vi "ABR-CPMR.vi"() -> ()   [LabVIEW 2014]
uses:
  <vilib>/DAQmx/create/channels.llb/DAQmx Create Channel (AI-Voltage-Basic).vi
  <vilib>/DAQmx/configure/trigger.llb/DAQmx Start Trigger (Digital Edge).vi
  <vilib>/DAQmx/create/channels.llb/DAQmx Create Channel (AO-Voltage-Basic).vi
  <vilib>/DAQmx/configure/timing.llb/DAQmx Timing (Sample Clock).vi
  <vilib>/DAQmx/write.llb/DAQmx Write (Analog Wfm 1Chan NSamp).vi
  <vilib>/DAQmx/read.llb/DAQmx Read (Analog Wfm 1Chan NSamp).vi
  <vilib>/measure/NI_MABase.lvlib
  <resource>/objmgr/daqmx.rc
panel:
  out "Averaged Acq Graph":waveform(dbl)(graph)
  out "C settings str":string[][](array[string])
  out "WN settings str":string[][](array[string])
  out "PT settings str":string[][](array[string])
  in  "Stop!":bool
  out "Expinfo words":string[](array[string])
  out "counter 2":i32
  out "First file array":bool[](array[boolean])
  out "Current test":i32(knob) scale=0.0..10.0
  out "Delay duration (ms)":dbl[](array[numeric])
  out "Stimulus duration (ms)":dbl[](array[numeric])
  out "Signal duration (ms)":dbl[](array[numeric])
  out "End of test":bool
  out "Stim file name":string[](array[string])
  out "Date_Time":string
  out "Main file name":string[](array[string])
  out "Fs":string
  out "File path str":string
  in  "Subject ID":string
  out "Expinfo name":string[](array[string])
  out "File name":string[](array[string])
  in  "File path":path
  in  "User name":string
  out "Group array settings":dbl[][](array[numeric])
  out "counter":i32
  in  "Start!":bool
  in  "Output Channel":tag="PXI1Slot6/ao0"
  out "Acquisition Graph":waveform(dbl)(graph)
  in  "Input Channel":tag="PXI1Slot6/ai0"
  out "Fs (#S/s)":dbl
  out "Stimulus Graph":waveform(dbl)(graph)
  out "iteration2":i32
  in  "Sampling info":cluster{"Fs (#S/s)":dbl, "#S":dbl}={"Fs (#S/s)"=100000.0, "#S"=200000.0}
  out "Protocol list":string[](array[string])
  out "Protocol array settings":dbl[][](array[numeric])
  out "C settings":dbl[](array[numeric])
  out "WN settings":dbl[](array[numeric])
  in  "Type of stimulus":u16(ring)=3 items=["Pure Tones", "White Noise", "Clic", "Choose..."]
  out "C words":string[](array[string])
  out "WN words":string[](array[string])
  out "iteration":i32
  in  "How many tests?":i32(slide)=1 scale=0.0..10.0
  out "PT words":string[](array[string])
  out "PT settings":dbl[](array[numeric])
  out "Tab Control":enum32{"Pure Tones", "White Noise", "Clic"}(tab)
  in  "Frequency (Hz)":u16(ring)=500 items=["500"=500, "1k"=1000, "2k"=2000, "4k"=4000, "8k"=8000, "16k"=16000, "32k"=32000, "40k"=40000]
  in  "Stimulation freq (stim/sec)":i32=20
  in  "Add Button":bool
  in  "Amplitude (dB SPL)":dbl=10.0 min=10.0 max=90.0 step=10.0
  in  "# Repetitions":u16(ring)=1000 items=["500"=500, "1000"=1000, "1500"=1500, "2000"=2000]
  in  "Amplitude (dB SPL)":dbl=30.0 min=10.0 max=90.0 step=10.0
  in  "Stimulation freq (stim/sec)":i32=20
  in  "Add Button":bool
  in  "# Repetitions":u16(ring)=1000 items=["500"=500, "1000"=1000, "1500"=1500, "2000"=2000]
  in  "Add Button":bool
  in  "Amplitude (dB SPL)":dbl=10.0 min=10.0 max=90.0 step=10.0
  in  "Stimulation freq (stim/sec)":i32=20
  in  "# Repetitions":u16(ring)=1000 items=["500"=500, "1000"=1000, "1500"=1500, "2000"=2000]
  # "Protocol list:"
  # "User, Subject and File settings:"
  # "Protocol settings:"
  # "1"
  # "(without spaces)"
  # "(without spaces)"
  # "4"
  # "(without spaces)"
  # "5"
  # "2"
  # "Choose channels:"
  # "6"
  # "3"
  # "Select sample rate:"
  # "Copyright 2016 División de Ciencias e Ingenierías, Campus León,\nUniversidad de Guanajuato\nPor: Cecilia Paulina Mares Román <cecypau.mr@gmail.com>"
  # "8"
  # "7"
  # "7"
  # "7"
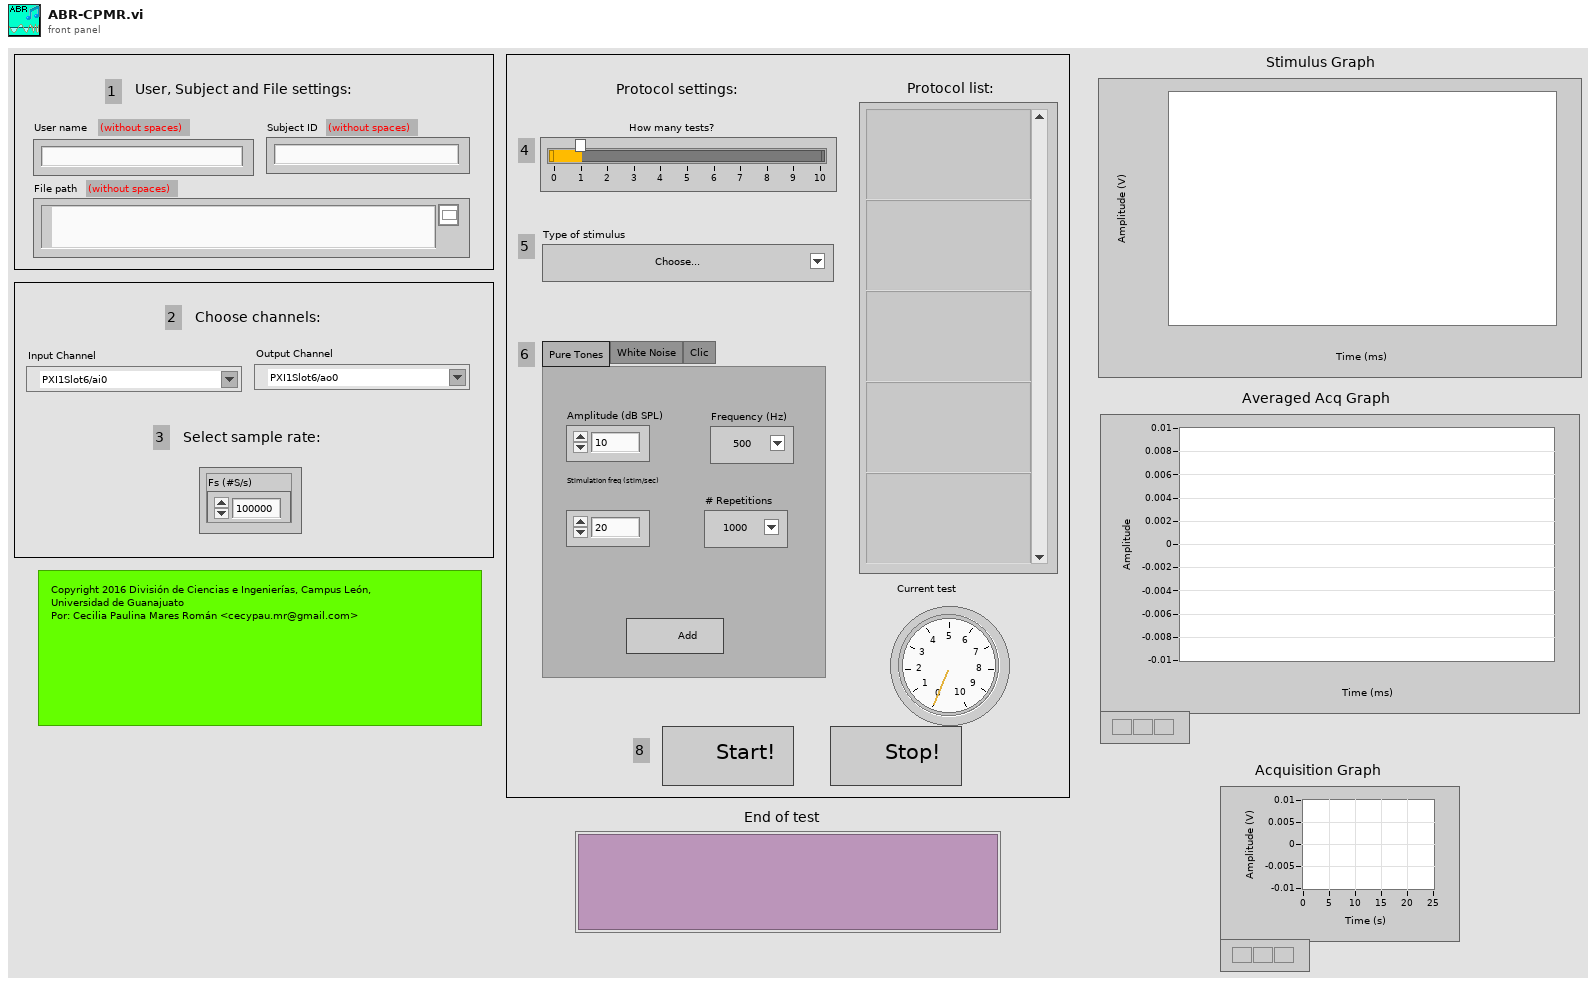
[diagram p1: front panel]
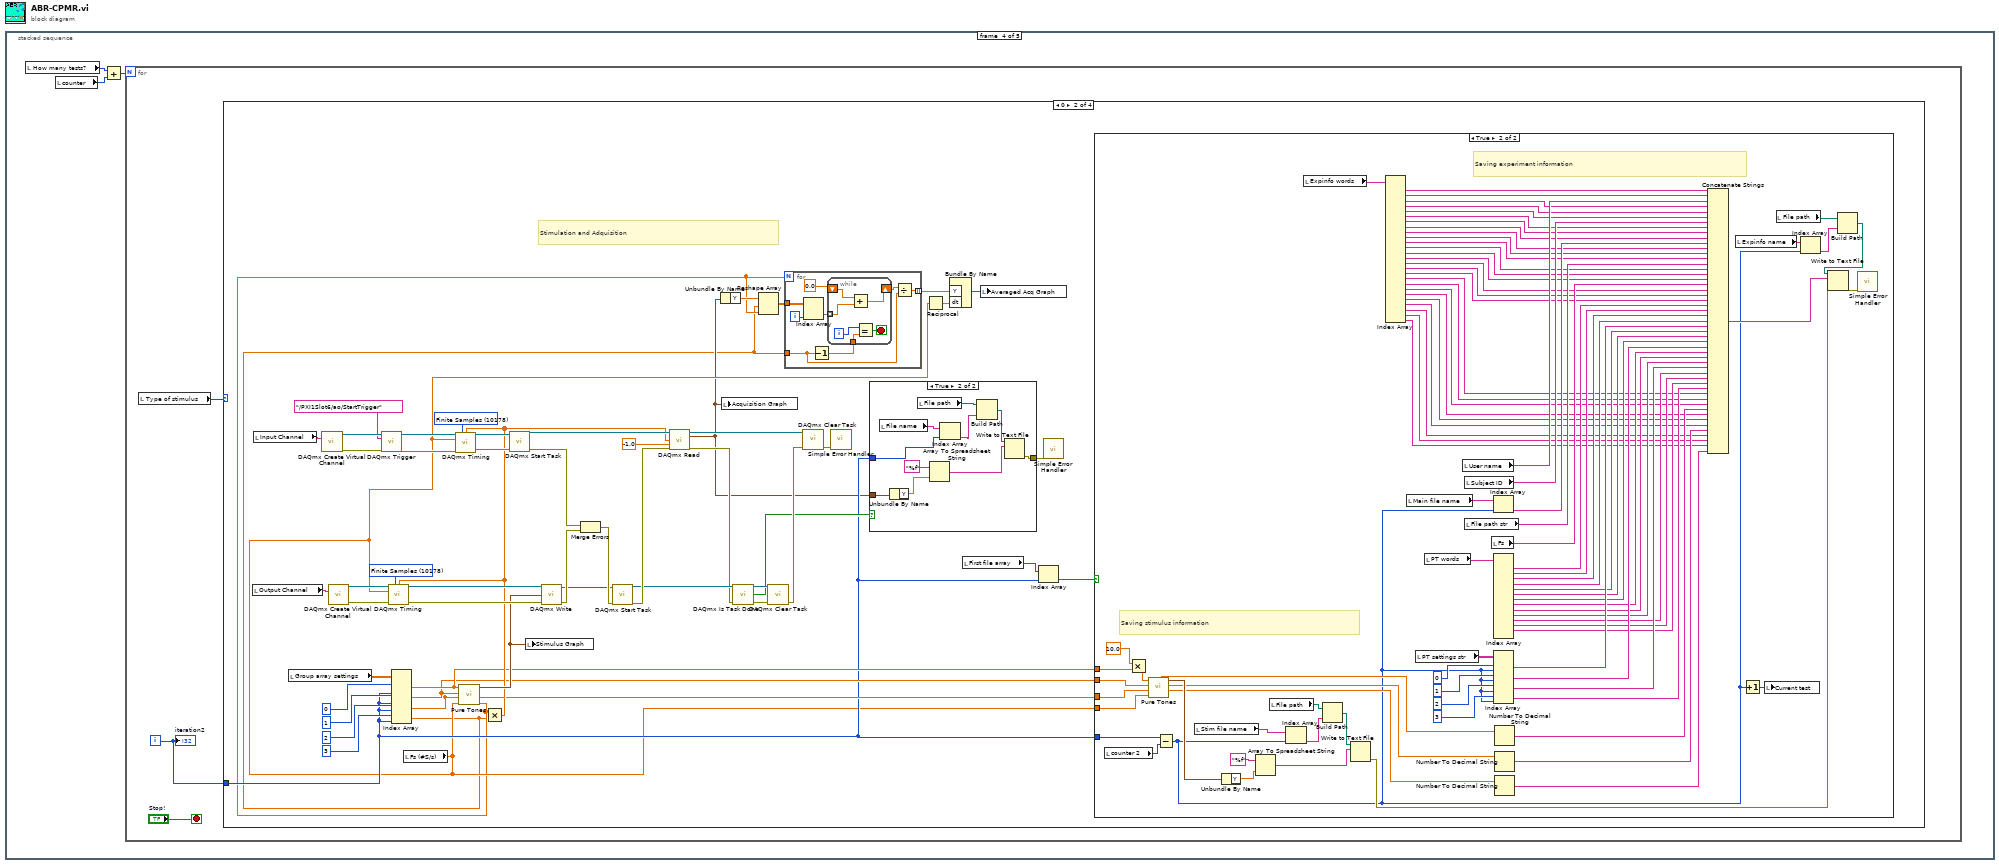
[diagram p0: block diagram]
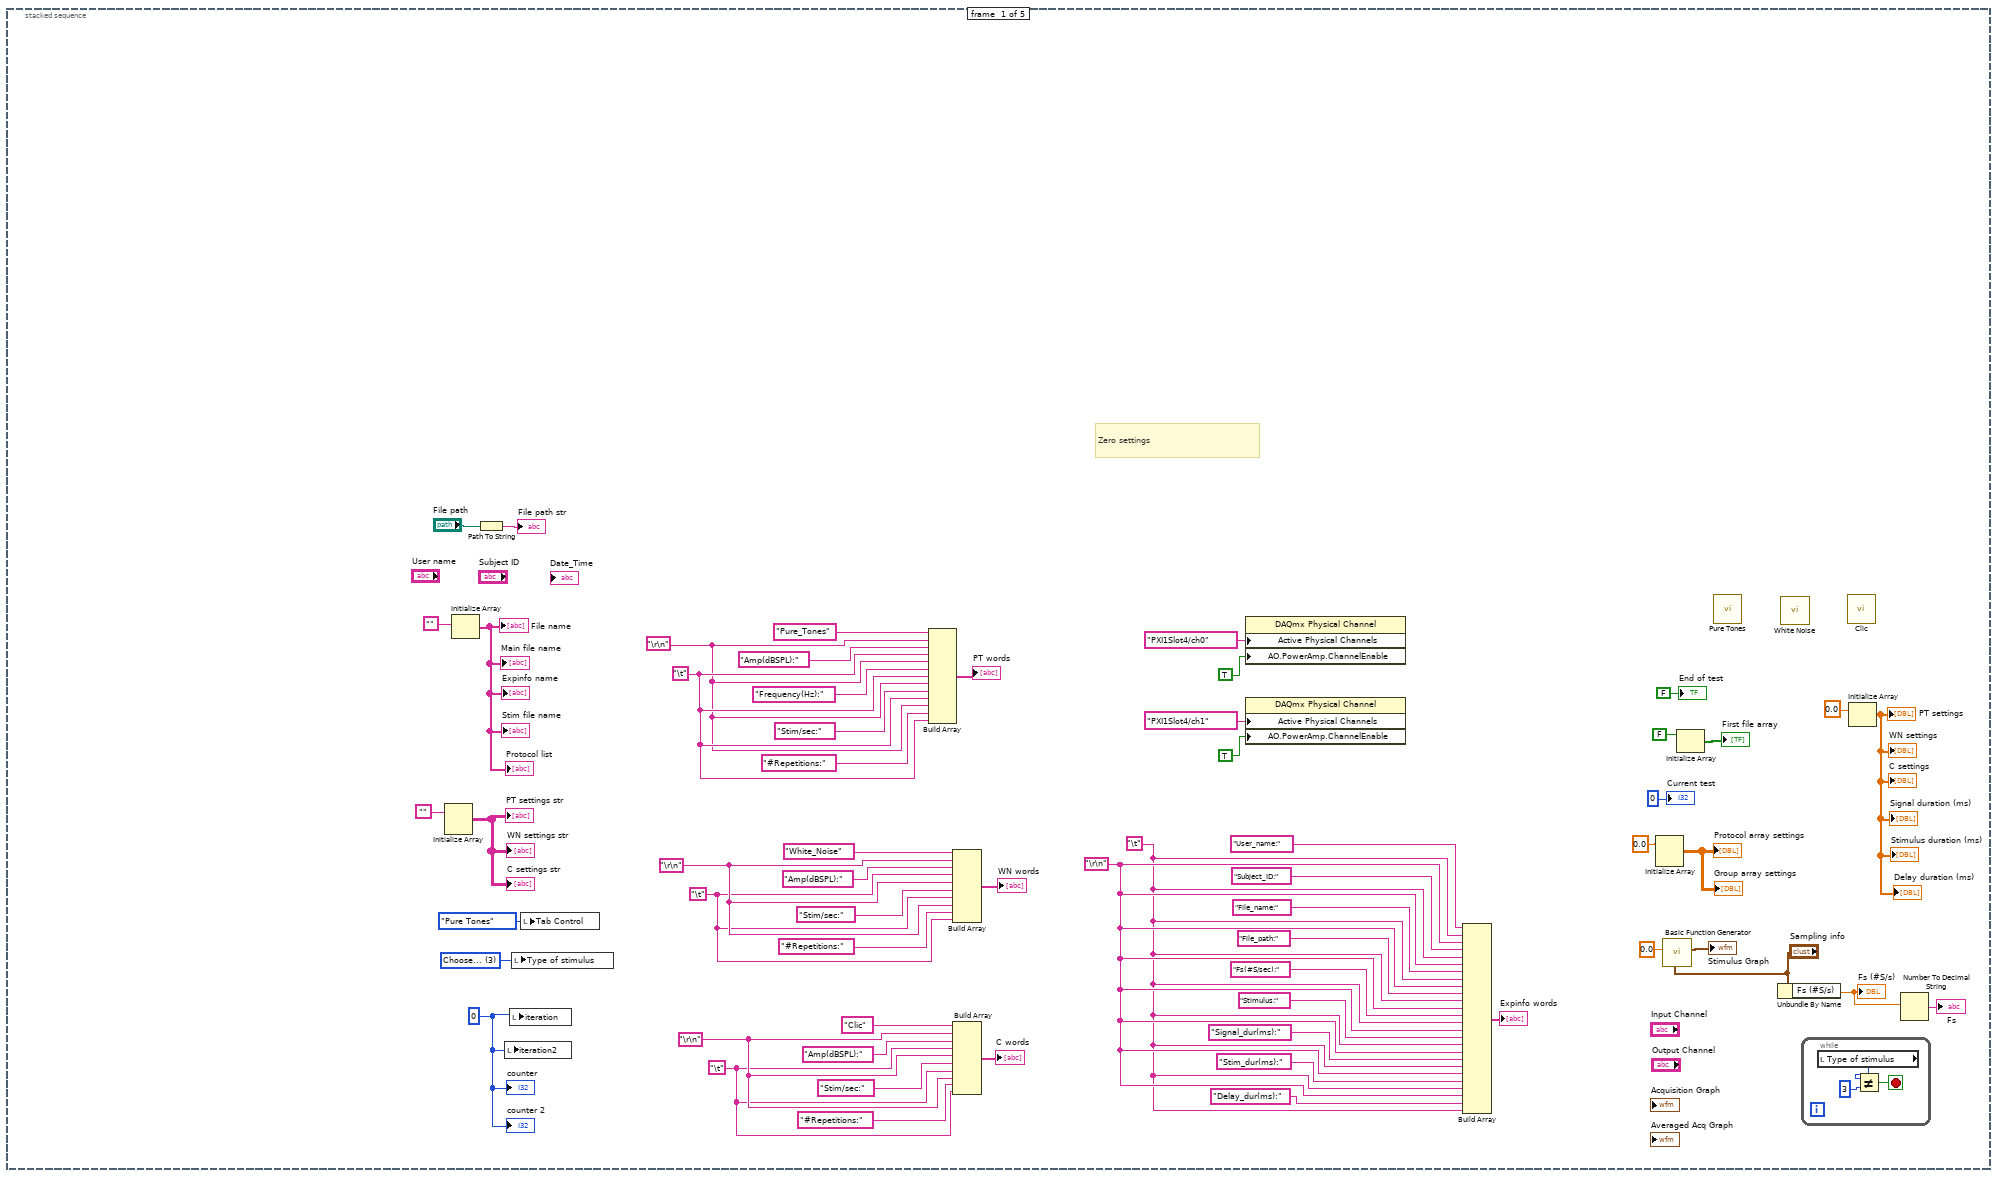
[diagram p2: hidden frame]
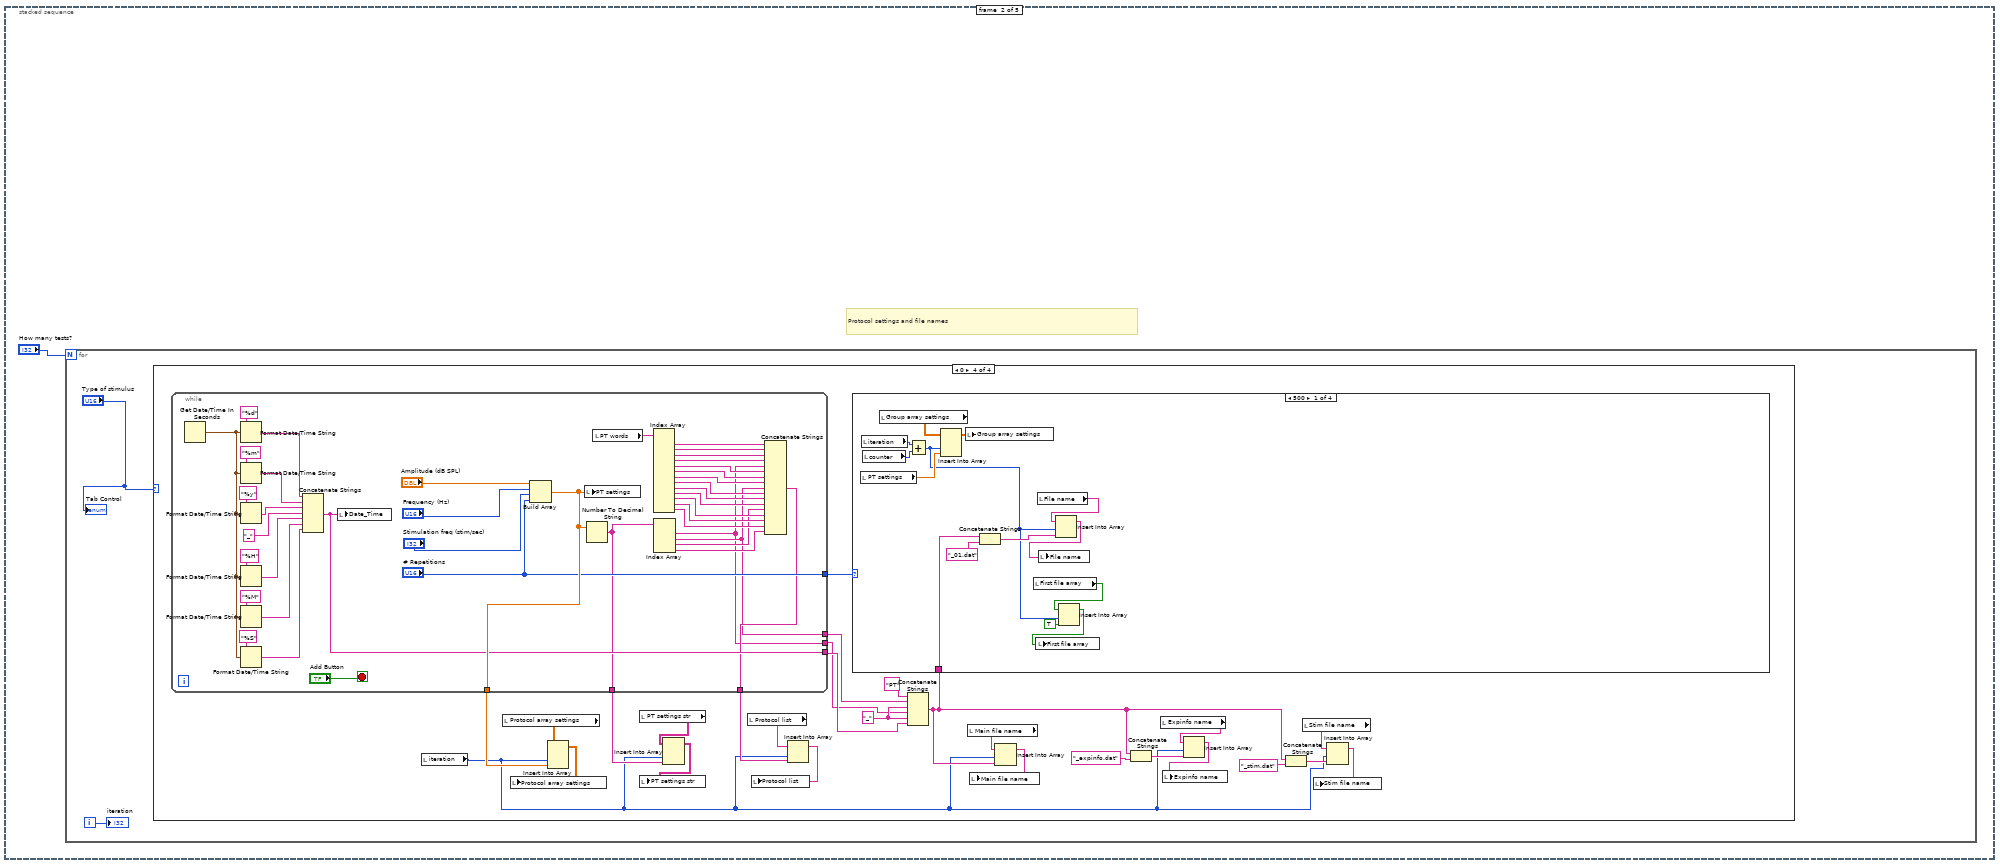
[diagram p3: hidden frame]
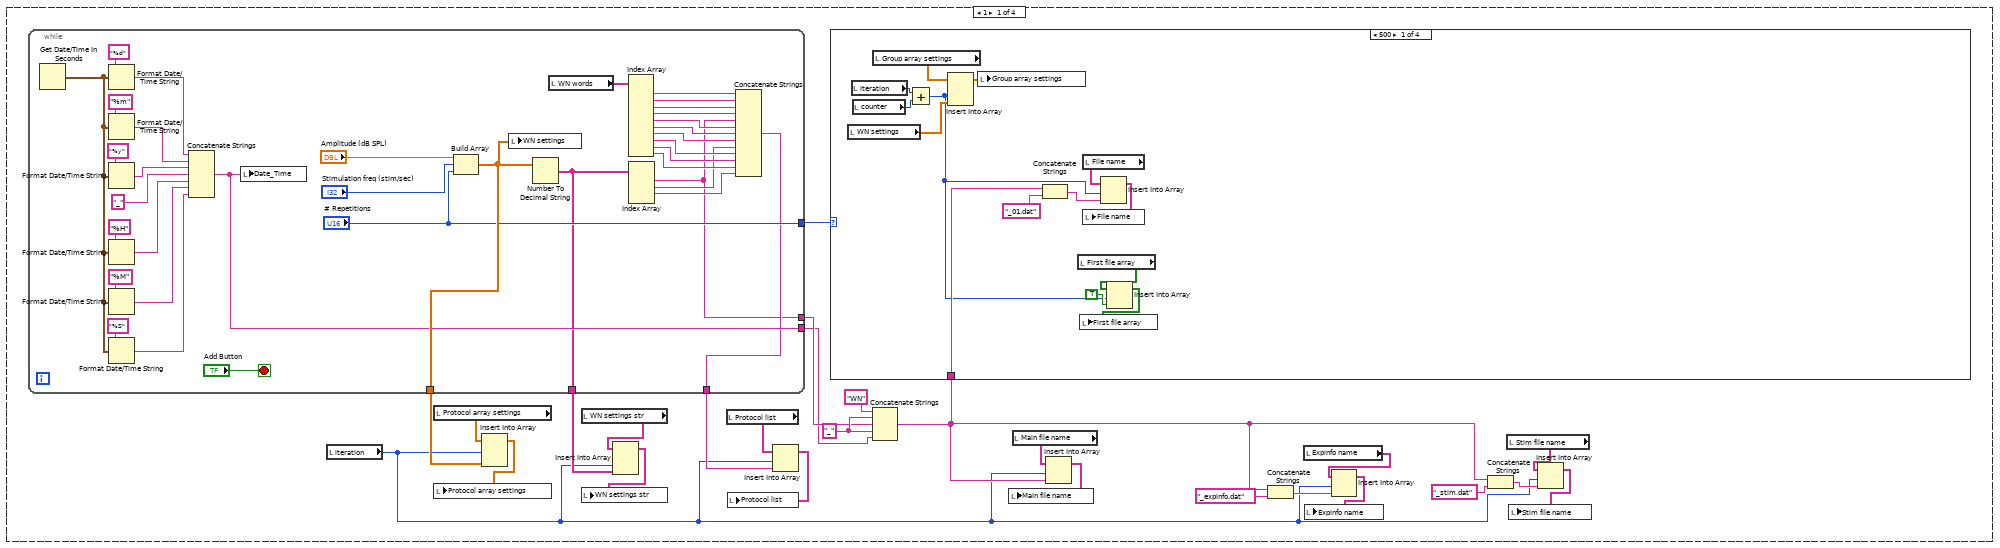
[diagram p4: hidden frame]
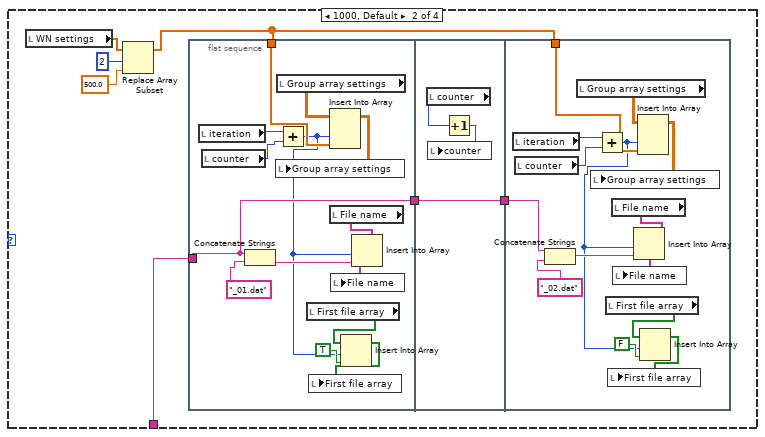
[diagram p5: hidden frame]
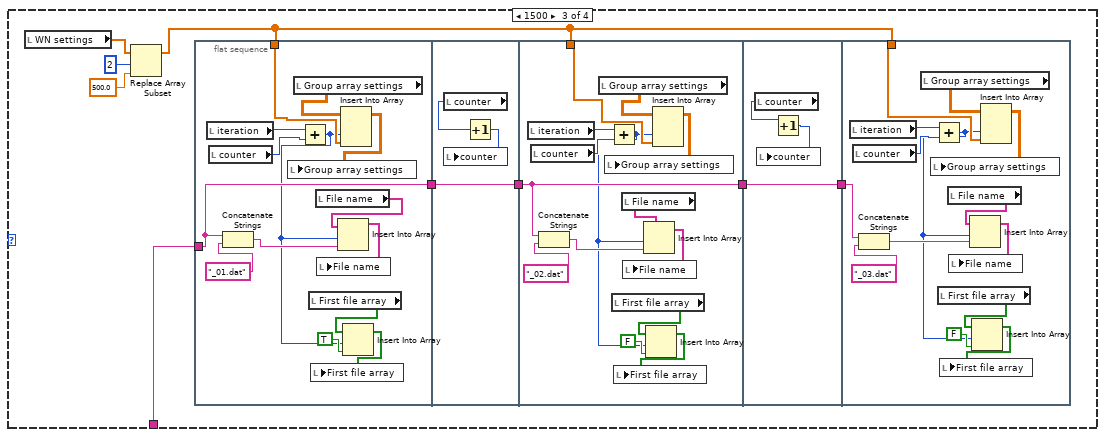
[diagram p6: hidden frame]
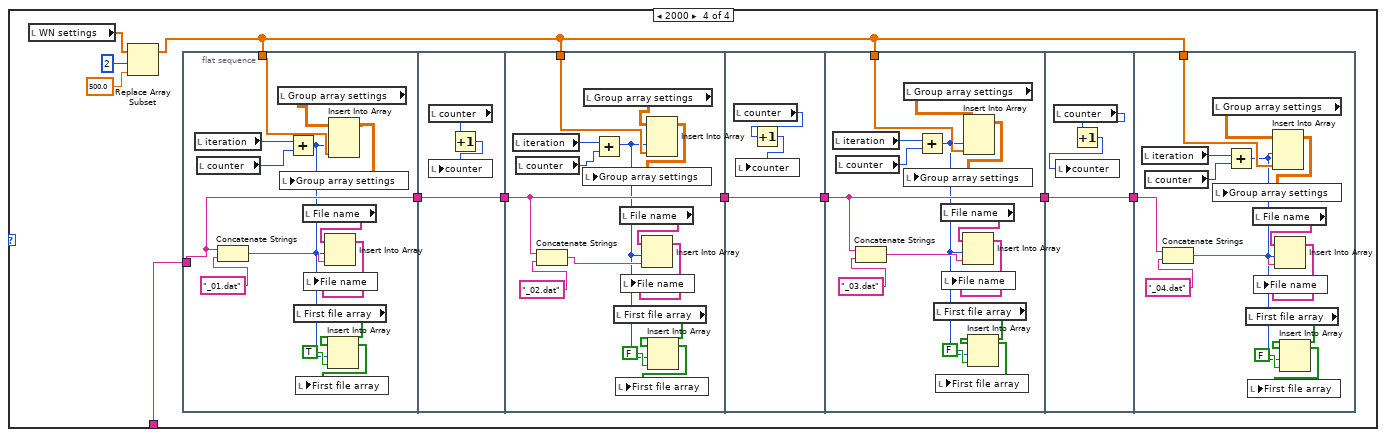
[diagram p7: hidden frame]
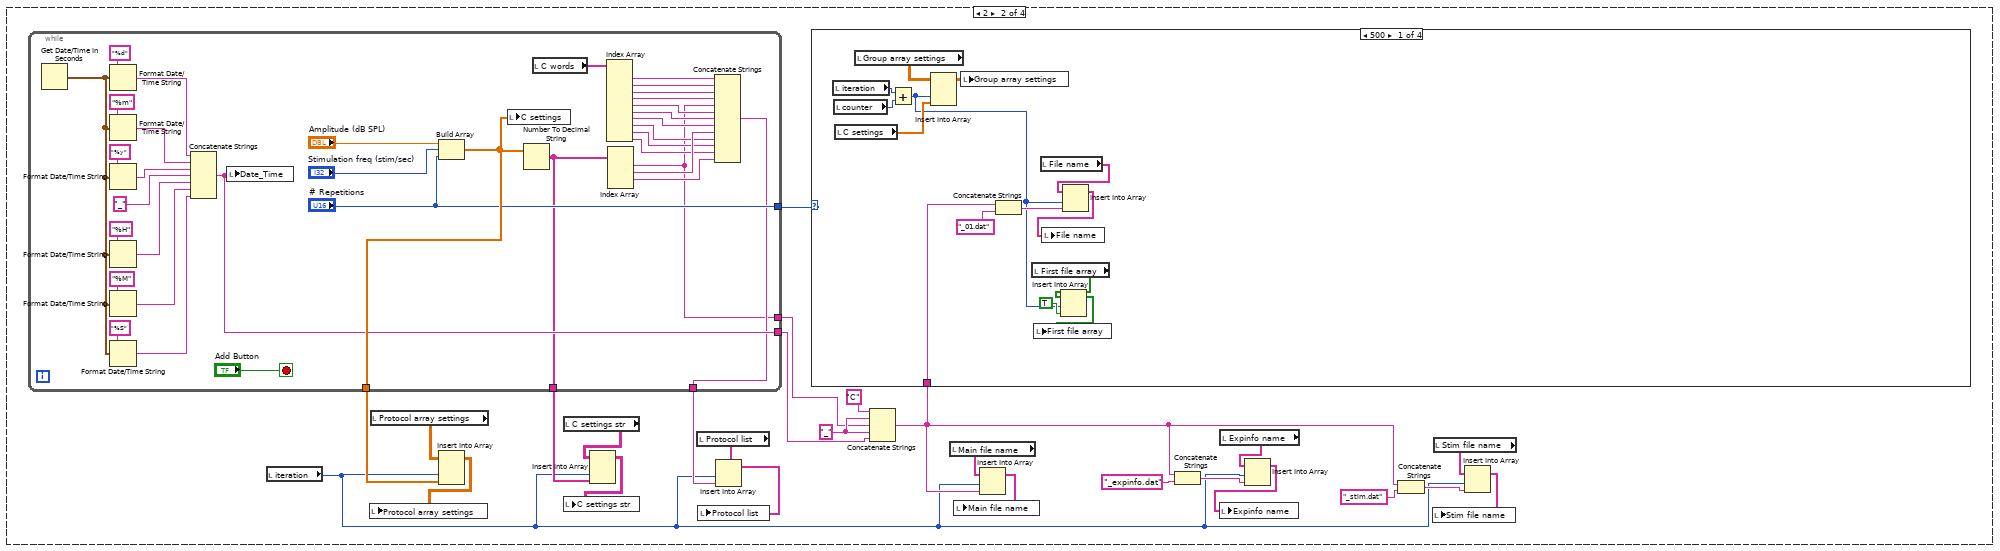
[diagram p8: hidden frame]
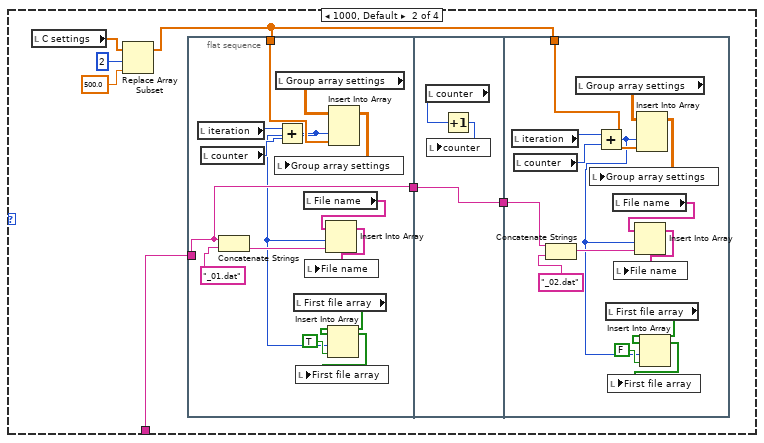
[diagram p9: hidden frame]
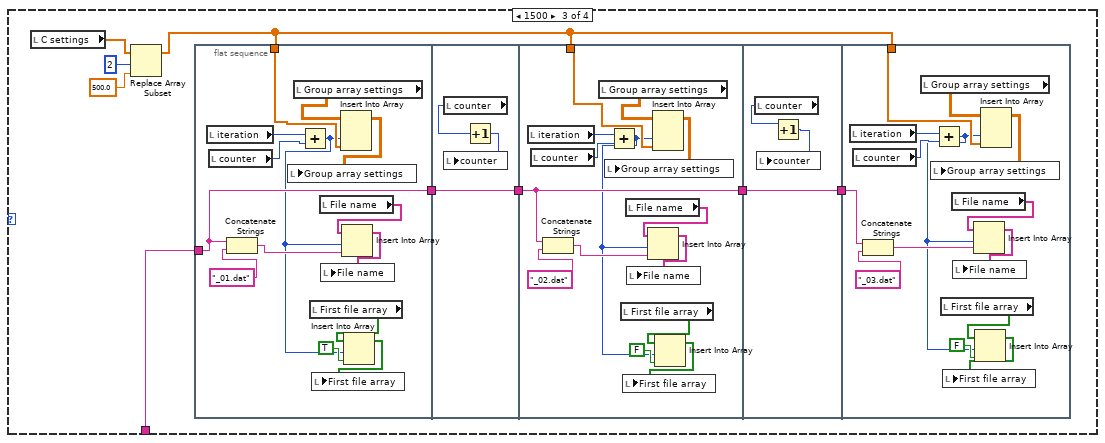
[diagram p10: hidden frame]
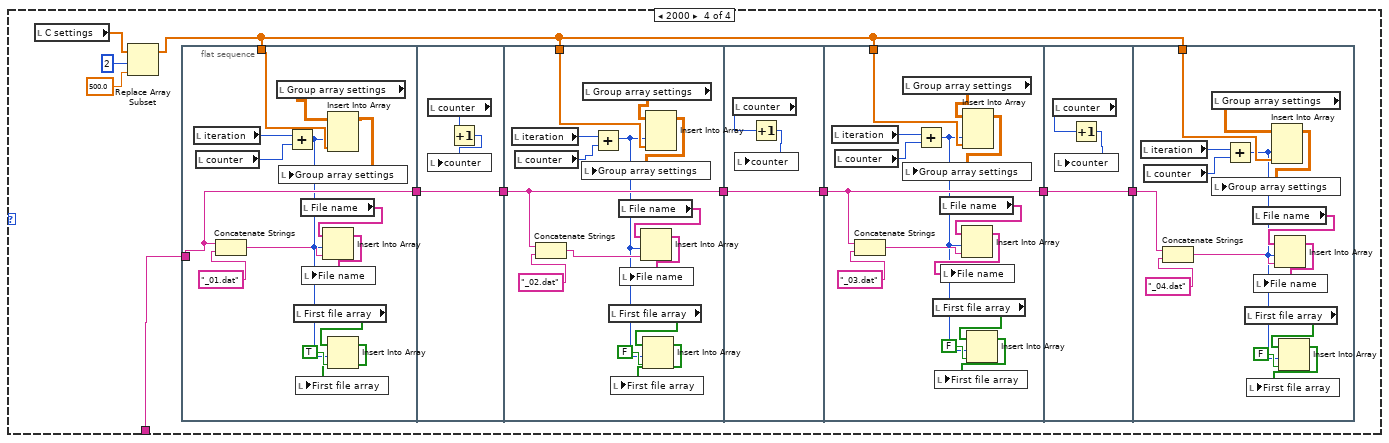
[diagram p11: hidden frame]
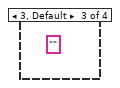
[diagram p12: hidden frame]
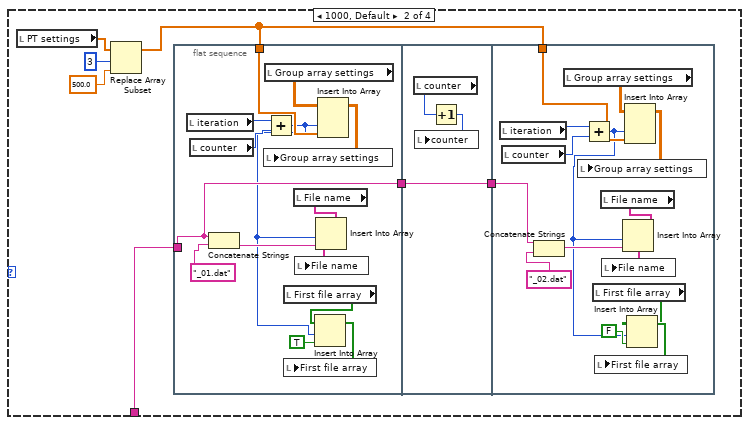
[diagram p13: hidden frame]
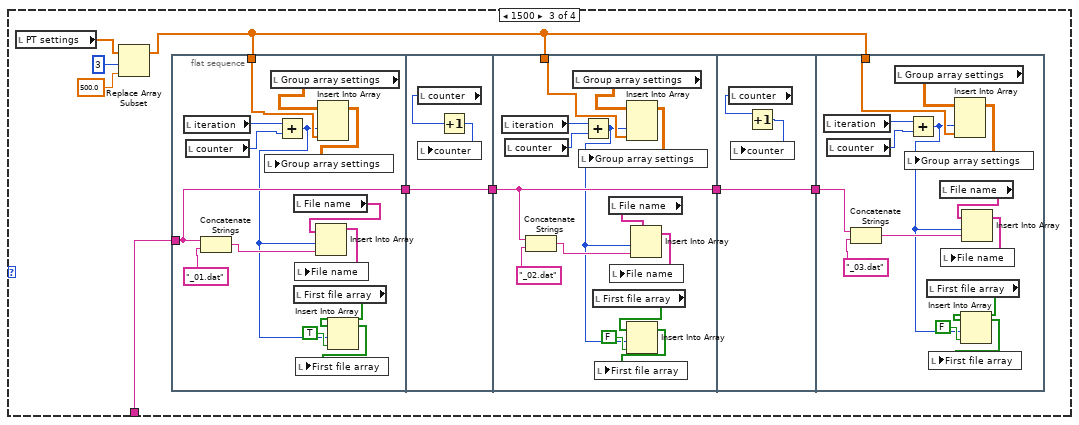
[diagram p14: hidden frame]
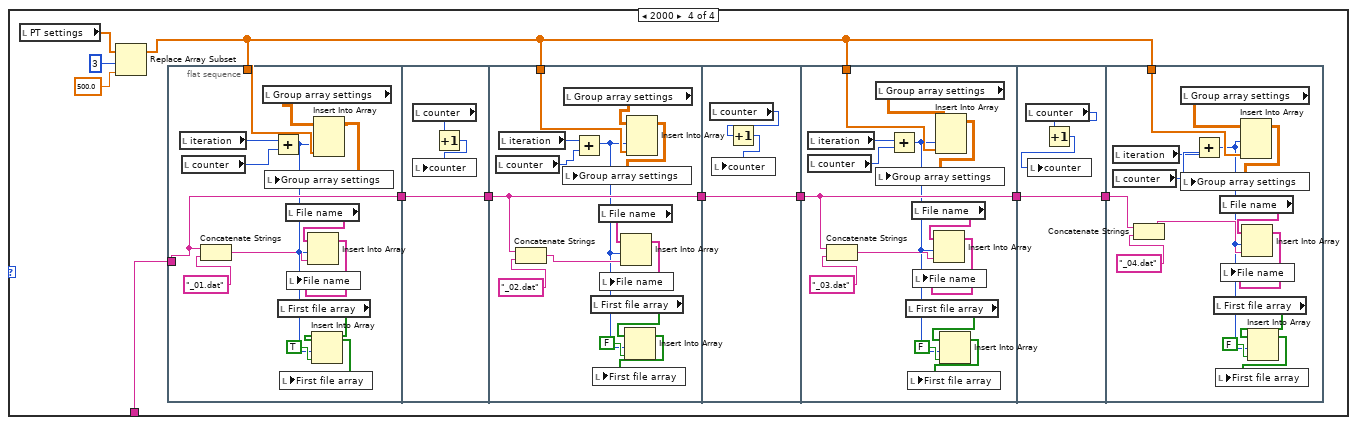
[diagram p15: hidden frame]
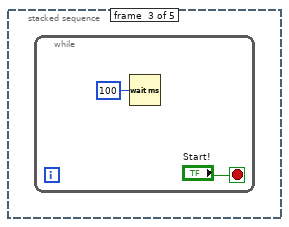
[diagram p16: hidden frame]
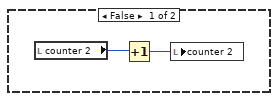
[diagram p18: hidden frame]
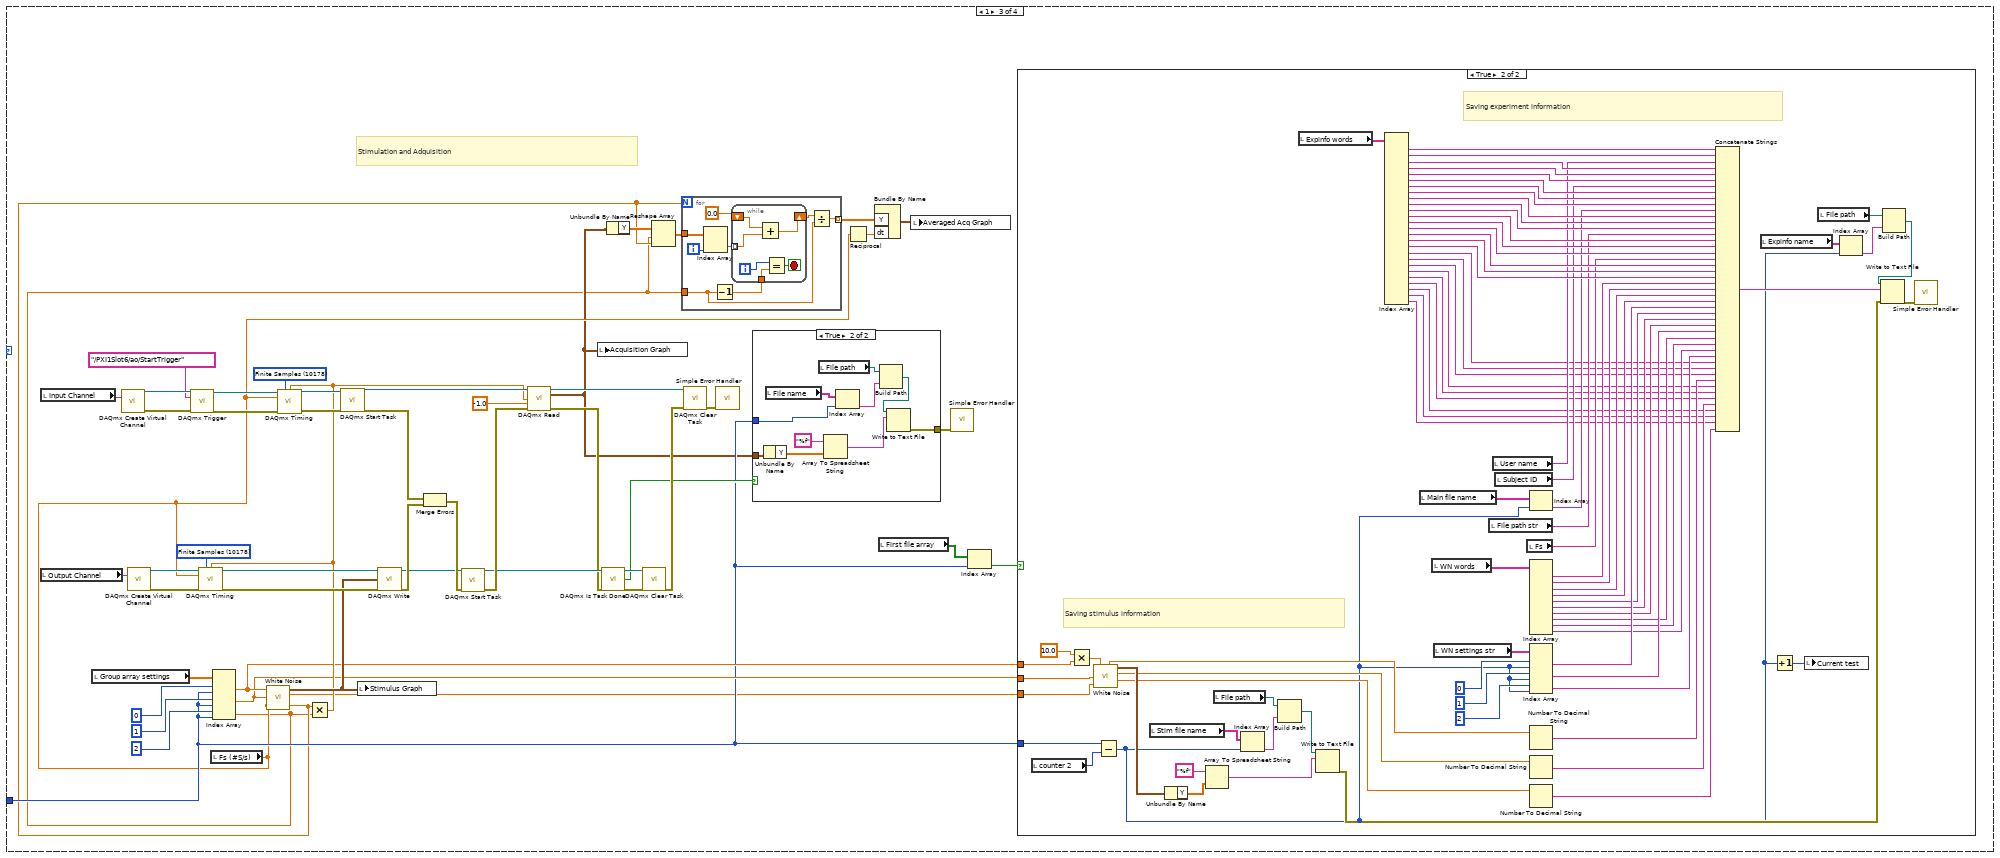
[diagram p20: hidden frame]
diagram:
  n1 = stacked-sequence {
    frame #0 {
      w16 = "\t"
      w18 = "\r\n"
      w20 = "\t"
      w22 = "\r\n"
      w26 = "\t"
      w28 = "\r\n"
      w33 = "\t"
      w32 = "\r\n"
      w58 = u16 3 items=["Pure Tones", "White Noise", "Clic", "Choose..."] ("Menu Ring")
      w5 = 0 ("iteration")
      # "Zero settings"
      n2 = Initialize Array("") -> (→"PT settings str" →"WN settings str" →"C settings str":string[][])  [unwired: 2 in]
      n3 = Initialize Array("") -> (→"Protocol list" →"File name" →"Expinfo name" →"Main file name" →"Stim file name":string[])  [unwired: 1 in]
      n4 = Path To String(path="File path") -> (string=→"File path str":string)
      n5 = local write "iteration2"(w5) -> ()
      n6 = local write "iteration"(w5) -> ()
      n7 = local write "Type of stimulus"(w58) -> ()
      n8 = local write "Tab Control"(enum32{"Pure Tones", "White Noise", "Clic"}."Pure Tones" ("Tab Control")) -> ()
      n9 = Build Array("Pure_Tones" ("string"), w32, "Amp(dBSPL):", w33, w32, "Frequency(Hz):" ("string"), w33, w32, "Stim/sec:" ("string"), w33, w32, "#Repetitions:" ("string"), w33) -> (→"PT words":string[])
      n10 = Build Array("White_Noise" ("string"), w28, "Amp(dBSPL):", w26, w28, "Stim/sec:" ("string"), w26, w28, "#Repetitions:" ("string"), w26) -> (→"WN words":string[])
      n11 = Build Array("Clic" ("string"), w22, "Amp(dBSPL):", w20, w22, "Stim/sec:" ("string"), w20, w22, "#Repetitions:" ("string"), w20) -> (→"C words":string[])
      n12 = property class="DAQmx Physical Channel"("Active Physical Channels"=tag "PXI1Slot4/ch0" ("ActivePhysicalChans"), "AO.PowerAmp.ChannelEnable"=TRUE) -> ()  [unwired: 2 in, 2 out]
      n13 = property class="DAQmx Physical Channel"("Active Physical Channels"=tag "PXI1Slot4/ch1" ("ActivePhysicalChans"), "AO.PowerAmp.ChannelEnable"=TRUE) -> ()  [unwired: 2 in, 2 out]
      n14 = Build Array("User_name:", w16, w18, "Subject_ID:", w16, w18, "File_name:", w16, w18, "File_path:", w16, w18, "Fs(#S/sec):", w16, w18, "Stimulus:", w16, w18, "Signal_dur(ms):", w16, w18, "Stim_dur(ms):", w16, w18, "Delay_dur(ms):", w16) -> (→"Expinfo words":string[])
      n15 = Initialize Array(0.0 ("element")) -> (→"Protocol array settings" →"Group array settings":dbl[][])  [unwired: 2 in]
      n16 = call <vilib>:"Basic Function Generator.vi"("sampling info"="Sampling info", "amplitude"=0.0) -> ("signal out"=→"Stimulus Graph":waveform(dbl))  [unwired: 7 in, 2 out]
      n17 = Initialize Array(FALSE) -> (→"First file array":bool[])  [unwired: 1 in]
      n18 = call <userlib>:"Pure Tones.vi"() -> ()  [unwired: 4 in, 5 out]
      n19 = Unbundle By Name("Sampling info") -> ("Fs (#S/s)"=w47:dbl)
      "Fs (#S/s)" <- w47
      n20 = call <userlib>:"White Noise.vi"() -> ()  [unwired: 3 in, 5 out]
      n21 = while {
        stop <- w61 stop-if-true
        n22 = local read "Type of stimulus"() -> (w63:u16)
        n23 = Not Equal?(x=w63, y=u16 3) -> (x != y?=w61:bool)
      }
      n24 = call <userlib>:"Clic.vi"() -> ()  [unwired: 3 in, 5 out]
      n25 = Initialize Array(0.0 ("element")) -> (→"C settings" →"PT settings" →"WN settings" →"Signal duration (ms)" →"Stimulus duration (ms)" →"Delay duration (ms)":dbl[])  [unwired: 1 in]
      n26 = Number To Decimal String(number=w47) -> (decimal integer string=→"Fs":string)  [unwired: 1 in]
      "counter" <- w5
      "End of test" <- FALSE ("End of test")
      "Current test" <- 0 ("Current test")
      "counter 2" <- w5
    }
    frame #1 {
      # "Protocol settings and file names"
      n27 = for {
        N: "How many tests?" -> [_]
        i -> [w66]
        n28 = case shown="0" "Type of stimulus" {
          frame 1 {
            w83 = "_"
            n29 = while {
              tunnel: [w280] -> w74
              tunnel: [w313] -> w92
              tunnel: ["# Repetitions"] -> w87
              tunnel: [w279] -> w73
              tunnel: [w297] -> w72
              tunnel: [w278] -> w68
              stop <- "Add Button" stop-if-true
              n30 = Get Date/Time In Seconds() -> (seconds since 1Jan1904=w305:timestamp)
              n31 = Format Date/Time String(time format string (%c)="%d", seconds (now)=w305) -> (date/time string=w304:string)  [unwired: 1 in]
              n32 = Format Date/Time String(time format string (%c)="%m", seconds (now)=w305) -> (date/time string=w303:string)  [unwired: 1 in]
              n33 = Format Date/Time String(time format string (%c)="%y", seconds (now)=w305) -> (date/time string=w302:string)  [unwired: 1 in]
              n34 = Format Date/Time String(time format string (%c)="%H", seconds (now)=w305) -> (date/time string=w301:string)  [unwired: 1 in]
              n35 = Format Date/Time String(time format string (%c)="%M", seconds (now)=w305) -> (date/time string=w300:string)  [unwired: 1 in]
              n36 = Format Date/Time String(time format string (%c)="%S", seconds (now)=w305) -> (date/time string=w299:string)  [unwired: 1 in]
              n37 = Concatenate Strings(w304, w303, w302, "_", w301, w300, w299) -> (w297:string)
              n38 = local write "Date_Time"(w297) -> ()
              n39 = Build Array("Amplitude (dB SPL)", "Stimulation freq (stim/sec)", "# Repetitions") -> (w313:dbl[])
              n40 = local write "WN settings"(w313) -> ()
              n41 = Number To Decimal String(number=w313) -> (decimal integer string=w278:string[])  [unwired: 1 in]
              n42 = local read "WN words"() -> (w281:string[])
              n43 = Index Array(array=w281) -> (element #1=w283:string, element #2=w284:string, element #3=w285:string, element #4=w286:string, element #5=w287:string, element #6=w288:string, element #7=w289:string, element #8=w290:string, element #9=w291:string, element #10=w292:string)  [unwired: 10 in]
              n44 = Index Array(array=w278) -> (element #1=w279:string, element #2=w282:string, element #3=w293:string)  [unwired: 4 in, 1 out]
              n45 = Concatenate Strings(w283, w284, w285, w286, w279, w287, w288, w289, w282, w290, w291, w292, w293) -> (w280:string)
            }
            n46 = local read "iteration"() -> (w67:i32)
            n47 = local read "Protocol array settings"() -> (w91:dbl[][])
            n48 = Insert Into Array(array=w91, index (col)=w67, new element=w92) -> (w90:dbl[][])  [unwired: 1 in]
            n49 = local write "Protocol array settings"(w90) -> ()
            n50 = local read "WN settings str"() -> (w69:string[][])
            n51 = Insert Into Array(array=w69, index (col)=w67, new element=w68) -> (w70:string[][])  [unwired: 1 in]
            n52 = local write "WN settings str"(w70) -> ()
            n53 = local read "Protocol list"() -> (w89:string[])
            n54 = Insert Into Array(array=w89, index=w67, new element=w74) -> (w88:string[])
            n55 = local write "Protocol list"(w88) -> ()
            n56 = Concatenate Strings("WN", w83, w73, w83, w72) -> (w71:string)
            n57 = case shown="500" w87 {
              tunnel: w71 -> [w97 w107 w145 w202]
              frame 500 {
                n58 = local read "WN settings"() -> (w106:dbl[])
                n59 = local read "iteration"() -> (w99:i32)
                n60 = local read "counter"() -> (w103:i32)
                n61 = local read "Group array settings"() -> (w105:dbl[][])
                n62 = Add(x=w99, y=w103) -> (x+y=w93:i32)
                n63 = Insert Into Array(array=w105, index (col)=w93, new element=w106) -> (w104:dbl[][])  [unwired: 1 in]
                n64 = local write "Group array settings"(w104) -> ()
                n65 = Concatenate Strings(w97, "_01.dat") -> (w98:string)
                n66 = local read "First file array"() -> (w94:bool[])
                n67 = local read "File name"() -> (w102:string[])
                n68 = Insert Into Array(array=w102, index=w93, new element=w98) -> (w101:string[])
                n69 = local write "File name"(w101) -> ()
                n70 = Insert Into Array(array=w94, index=w93, new element=TRUE) -> (w95:bool[])
                n71 = local write "First file array"(w95) -> ()
              }
              frame 1000, Default {
                n72 = local read "WN settings"() -> (w113:dbl[])
                n73 = Replace Array Subset(array=w113, new element=500.0 ("new element/subarray"), index=2) -> (w108:dbl[])
                n74 = flat-sequence {
                  tunnel: w108 -> [w125]
                  tunnel: w107 -> [w118]
                  tunnel: [w118] -> w109
                  tunnel: [w128] -> w110
                  tunnel: w109 -> [w128]
                  tunnel: w108 -> [w140]
                  tunnel: w110 -> [w139]
                  frame #0 {
                    n75 = local read "iteration"() -> (w124:i32)
                    n76 = local read "counter"() -> (w123:i32)
                    n77 = Concatenate Strings(w118, "_01.dat") -> (w119:string)
                    n78 = local read "Group array settings"() -> (w126:dbl[][])
                    n79 = Add(x=w124, y=w123) -> (x+y=w114:i32)
                    n80 = local read "First file array"() -> (w115:bool[])
                    n81 = Insert Into Array(array=w126, index (col)=w114, new element=w125) -> (w127:dbl[][])  [unwired: 1 in]
                    n82 = local write "Group array settings"(w127) -> ()
                    n83 = local read "File name"() -> (w121:string[])
                    n84 = Insert Into Array(array=w115, index=w114, new element=TRUE) -> (w116:bool[])
                    n85 = local write "First file array"(w116) -> ()
                    n86 = Insert Into Array(array=w121, index=w114, new element=w119) -> (w120:string[])
                    n87 = local write "File name"(w120) -> ()
                  }
                  frame #1 {
                    n88 = local read "counter"() -> (w130:i32)
                    n89 = Increment(x=w130) -> (x+1=w129:i32)
                    n90 = local write "counter"(w129) -> ()
                  }
                  frame #2 {
                    n91 = local read "iteration"() -> (w141:i32)
                    n92 = local read "counter"() -> (w142:i32)
                    n93 = Concatenate Strings(w139, "_02.dat") -> (w135:string)
                    n94 = local read "Group array settings"() -> (w143:dbl[][])
                    n95 = Add(x=w141, y=w142) -> (x+y=w132:i32)
                    n96 = local read "First file array"() -> (w133:bool[])
                    n97 = local read "File name"() -> (w137:string[])
                    n98 = Insert Into Array(array=w137, index=w132, new element=w135) -> (w136:string[])
                    n99 = local write "File name"(w136) -> ()
                    n100 = Insert Into Array(array=w143, index (col)=w132, new element=w140) -> (w144:dbl[][])  [unwired: 1 in]
                    n101 = local write "Group array settings"(w144) -> ()
                    n102 = Insert Into Array(array=w133, index=w132, new element=FALSE) -> (w131:bool[])
                    n103 = local write "First file array"(w131) -> ()
                  }
                }
              }
              frame 1500 {
                n104 = local read "WN settings"() -> (w151:dbl[])
                n105 = Replace Array Subset(array=w151, new element=500.0 ("new element/subarray"), index=2) -> (w146:dbl[])
                n106 = flat-sequence {
                  tunnel: w146 -> [w163]
                  tunnel: w145 -> [w158]
                  tunnel: [w158] -> w147
                  tunnel: [w168] -> w150
                  tunnel: w147 -> [w168]
                  tunnel: w146 -> [w175]
                  tunnel: w150 -> [w179]
                  tunnel: [w179] -> w149
                  tunnel: w149 -> [w185]
                  tunnel: [w185] -> w148
                  tunnel: w146 -> [w197]
                  tunnel: w148 -> [w196]
                  frame #0 {
                    n107 = local read "iteration"() -> (w165:i32)
                    n108 = local read "counter"() -> (w164:i32)
                    n109 = Concatenate Strings(w158, "_01.dat") -> (w160:string)
                    n110 = local read "Group array settings"() -> (w167:dbl[][])
                    n111 = Add(x=w165, y=w164) -> (x+y=w155:i32)
                    n112 = local read "First file array"() -> (w156:bool[])
                    n113 = local read "File name"() -> (w159:string[])
                    n114 = Insert Into Array(array=w159, index=w155, new element=w160) -> (w162:string[])
                    n115 = local write "File name"(w162) -> ()
                    n116 = Insert Into Array(array=w167, index (col)=w155, new element=w163) -> (w166:dbl[][])  [unwired: 1 in]
                    n117 = local write "Group array settings"(w166) -> ()
                    n118 = Insert Into Array(array=w156, index=w155, new element=TRUE) -> (w154:bool[])
                    n119 = local write "First file array"(w154) -> ()
                  }
                  frame #1 {
                    n120 = local read "counter"() -> (w170:i32)
                    n121 = Increment(x=w170) -> (x+1=w169:i32)
                    n122 = local write "counter"(w169) -> ()
                  }
                  frame #2 {
                    n123 = local read "iteration"() -> (w182:i32)
                    n124 = local read "counter"() -> (w176:i32)
                    n125 = Concatenate Strings(w179, "_02.dat") -> (w177:string)
                    n126 = local read "Group array settings"() -> (w183:dbl[][])
                    n127 = Add(x=w182, y=w176) -> (x+y=w171:i32)
                    n128 = local read "First file array"() -> (w172:bool[])
                    n129 = local read "File name"() -> (w181:string[])
                    n130 = Insert Into Array(array=w181, index=w171, new element=w177) -> (w180:string[])
                    n131 = local write "File name"(w180) -> ()
                    n132 = Insert Into Array(array=w172, index=w171, new element=FALSE) -> (w173:bool[])
                    n133 = local write "First file array"(w173) -> ()
                    n134 = Insert Into Array(array=w183, index (col)=w171, new element=w175) -> (w184:dbl[][])  [unwired: 1 in]
                    n135 = local write "Group array settings"(w184) -> ()
                  }
                  frame #3 {
                    n136 = local read "counter"() -> (w186:i32)
                    n137 = Increment(x=w186) -> (x+1=w187:i32)
                    n138 = local write "counter"(w187) -> ()
                  }
                  frame #4 {
                    n139 = local read "iteration"() -> (w199:i32)
                    n140 = local read "counter"() -> (w198:i32)
                    n141 = Concatenate Strings(w196, "_03.dat") -> (w192:string)
                    n142 = local read "Group array settings"() -> (w200:dbl[][])
                    n143 = Add(x=w199, y=w198) -> (x+y=w188:i32)
                    n144 = local read "First file array"() -> (w189:bool[])
                    n145 = local read "File name"() -> (w195:string[])
                    n146 = Insert Into Array(array=w195, index=w188, new element=w192) -> (w194:string[])
                    n147 = local write "File name"(w194) -> ()
                    n148 = Insert Into Array(array=w189, index=w188, new element=FALSE) -> (w190:bool[])
                    n149 = local write "First file array"(w190) -> ()
                    n150 = Insert Into Array(array=w200, index (col)=w188, new element=w197) -> (w201:dbl[][])  [unwired: 1 in]
                    n151 = local write "Group array settings"(w201) -> ()
                  }
                }
              }
              frame 2000 {
                n152 = local read "WN settings"() -> (w210:dbl[])
                n153 = Replace Array Subset(array=w210, new element=500.0 ("new element/subarray"), index=2) -> (w203:dbl[])
                n154 = flat-sequence {
                  tunnel: w203 -> [w222]
                  tunnel: w202 -> [w217]
                  tunnel: [w217] -> w208
                  tunnel: [w227] -> w209
                  tunnel: w208 -> [w227]
                  tunnel: w203 -> [w236]
                  tunnel: w209 -> [w235]
                  tunnel: [w235] -> w207
                  tunnel: w207 -> [w244]
                  tunnel: [w244] -> w206
                  tunnel: w203 -> [w258]
                  tunnel: w206 -> [w255]
                  tunnel: [w255] -> w205
                  tunnel: w205 -> [w261]
                  tunnel: [w261] -> w204
                  tunnel: w203 -> [w273]
                  tunnel: w204 -> [w272]
                  frame #0 {
                    n155 = local read "iteration"() -> (w224:i32)
                    n156 = local read "counter"() -> (w223:i32)
                    n157 = Concatenate Strings(w217, "_01.dat") -> (w218:string)
                    n158 = local read "Group array settings"() -> (w226:dbl[][])
                    n159 = Add(x=w224, y=w223) -> (x+y=w213:i32)
                    n160 = local read "First file array"() -> (w214:bool[])
                    n161 = local read "File name"() -> (w219:string[])
                    n162 = Insert Into Array(array=w219, index=w213, new element=w218) -> (w220:string[])
                    n163 = local write "File name"(w220) -> ()
                    n164 = Insert Into Array(array=w214, index=w213, new element=TRUE) -> (w215:bool[])
                    n165 = local write "First file array"(w215) -> ()
                    n166 = Insert Into Array(array=w226, index (col)=w213, new element=w222) -> (w225:dbl[][])  [unwired: 1 in]
                    n167 = local write "Group array settings"(w225) -> ()
                  }
                  frame #1 {
                    n168 = local read "counter"() -> (w229:i32)
                    n169 = Increment(x=w229) -> (x+1=w228:i32)
                    n170 = local write "counter"(w228) -> ()
                  }
                  frame #2 {
                    n171 = local read "iteration"() -> (w234:i32)
                    n172 = local read "counter"() -> (w243:i32)
                    n173 = Concatenate Strings(w235, "_02.dat") -> (w239:string)
                    n174 = local read "Group array settings"() -> (w238:dbl[][])
                    n175 = Add(x=w234, y=w243) -> (x+y=w230:i32)
                    n176 = local read "First file array"() -> (w231:bool[])
                    n177 = local read "File name"() -> (w241:string[])
                    n178 = Insert Into Array(array=w241, index=w230, new element=w239) -> (w240:string[])
                    n179 = local write "File name"(w240) -> ()
                    n180 = Insert Into Array(array=w238, index (col)=w230, new element=w236) -> (w237:dbl[][])  [unwired: 1 in]
                    n181 = local write "Group array settings"(w237) -> ()
                    n182 = Insert Into Array(array=w231, index=w230, new element=FALSE) -> (w232:bool[])
                    n183 = local write "First file array"(w232) -> ()
                  }
                  frame #3 {
                    n184 = local read "counter"() -> (w246:i32)
                    n185 = Increment(x=w246) -> (x+1=w245:i32)
                    n186 = local write "counter"(w245) -> ()
                  }
                  frame #4 {
                    n187 = local read "iteration"() -> (w251:i32)
                    n188 = local read "counter"() -> (w256:i32)
                    n189 = Concatenate Strings(w255, "_03.dat") -> (w252:string)
                    n190 = local read "Group array settings"() -> (w260:dbl[][])
                    n191 = Add(x=w251, y=w256) -> (x+y=w247:i32)
                    n192 = local read "First file array"() -> (w248:bool[])
                    n193 = local read "File name"() -> (w254:string[])
                    n194 = Insert Into Array(array=w254, index=w247, new element=w252) -> (w253:string[])
                    n195 = local write "File name"(w253) -> ()
                    n196 = Insert Into Array(array=w260, index (col)=w247, new element=w258) -> (w257:dbl[][])  [unwired: 1 in]
                    n197 = local write "Group array settings"(w257) -> ()
                    n198 = Insert Into Array(array=w248, index=w247, new element=FALSE) -> (w249:bool[])
                    n199 = local write "First file array"(w249) -> ()
                  }
                  frame #5 {
                    n200 = local read "counter"() -> (w262:i32)
                    n201 = Increment(x=w262) -> (x+1=w263:i32)
                    n202 = local write "counter"(w263) -> ()
                  }
                  frame #6 {
                    n203 = local read "iteration"() -> (w268:i32)
                    n204 = local read "counter"() -> (w275:i32)
                    n205 = Concatenate Strings(w272, "_04.dat") -> (w269:string)
                    n206 = local read "Group array settings"() -> (w277:dbl[][])
                    n207 = Add(x=w268, y=w275) -> (x+y=w264:i32)
                    n208 = local read "First file array"() -> (w265:bool[])
                    n209 = local read "File name"() -> (w271:string[])
                    n210 = Insert Into Array(array=w277, index (col)=w264, new element=w273) -> (w274:dbl[][])  [unwired: 1 in]
                    n211 = local write "Group array settings"(w274) -> ()
                    n212 = Insert Into Array(array=w271, index=w264, new element=w269) -> (w270:string[])
                    n213 = local write "File name"(w270) -> ()
                    n214 = Insert Into Array(array=w265, index=w264, new element=FALSE) -> (w266:bool[])
                    n215 = local write "First file array"(w266) -> ()
                  }
                }
              }
            }
            n216 = local read "Main file name"() -> (w76:string[])
            n217 = Insert Into Array(array=w76, index=w67, new element=w71) -> (w75:string[])
            n218 = local write "Main file name"(w75) -> ()
            n219 = Concatenate Strings(w71, "_expinfo.dat") -> (w81:string)
            n220 = local read "Expinfo name"() -> (w85:string[])
            n221 = Insert Into Array(array=w85, index=w67, new element=w81) -> (w84:string[])
            n222 = local write "Expinfo name"(w84) -> ()
            n223 = Concatenate Strings(w71, "_stim.dat") -> (w79:string)
            n224 = local read "Stim file name"() -> (w78:string[])
            n225 = Insert Into Array(array=w78, index=w67, new element=w79) -> (w77:string[])
            n226 = local write "Stim file name"(w77) -> ()
          }
          frame 2 {
            w330 = "_"
            n227 = while {
              tunnel: [w559] -> w339
              tunnel: ["# Repetitions"] -> w334
              tunnel: [w526] -> w320
              tunnel: [w542] -> w318
              tunnel: [w527] -> w323
              tunnel: [w525] -> w315
              stop <- "Add Button" stop-if-true
              n228 = Get Date/Time In Seconds() -> (seconds since 1Jan1904=w550:timestamp)
              n229 = Format Date/Time String(time format string (%c)="%d", seconds (now)=w550) -> (date/time string=w549:string)  [unwired: 1 in]
              n230 = Format Date/Time String(time format string (%c)="%m", seconds (now)=w550) -> (date/time string=w548:string)  [unwired: 1 in]
              n231 = Format Date/Time String(time format string (%c)="%y", seconds (now)=w550) -> (date/time string=w547:string)  [unwired: 1 in]
              n232 = Format Date/Time String(time format string (%c)="%H", seconds (now)=w550) -> (date/time string=w546:string)  [unwired: 1 in]
              n233 = Format Date/Time String(time format string (%c)="%M", seconds (now)=w550) -> (date/time string=w545:string)  [unwired: 1 in]
              n234 = Format Date/Time String(time format string (%c)="%S", seconds (now)=w550) -> (date/time string=w544:string)  [unwired: 1 in]
              n235 = Concatenate Strings(w549, w548, w547, "_", w546, w545, w544) -> (w542:string)
              n236 = local write "Date_Time"(w542) -> ()
              n237 = Build Array("Amplitude (dB SPL)", "Stimulation freq (stim/sec)", "# Repetitions") -> (w559:dbl[])
              n238 = local write "C settings"(w559) -> ()
              n239 = Number To Decimal String(number=w559) -> (decimal integer string=w525:string[])  [unwired: 1 in]
              n240 = local read "C words"() -> (w540:string[])
              n241 = Index Array(array=w540) -> (element #1=w538:string, element #2=w537:string, element #3=w536:string, element #4=w535:string, element #5=w534:string, element #6=w533:string, element #7=w532:string, element #8=w531:string, element #9=w530:string, element #10=w529:string)  [unwired: 10 in]
              n242 = Index Array(array=w525) -> (element #1=w526:string, element #2=w539:string, element #3=w528:string)  [unwired: 4 in, 1 out]
              n243 = Concatenate Strings(w538, w537, w536, w535, w526, w534, w533, w532, w539, w531, w530, w529, w528) -> (w527:string)
            }
            n244 = local read "iteration"() -> (w314:i32)
            n245 = local read "Protocol array settings"() -> (w338:dbl[][])
            n246 = Insert Into Array(array=w338, index (col)=w314, new element=w339) -> (w337:dbl[][])  [unwired: 1 in]
            n247 = local write "Protocol array settings"(w337) -> ()
            n248 = local read "C settings str"() -> (w316:string[][])
            n249 = Insert Into Array(array=w316, index (col)=w314, new element=w315) -> (w317:string[][])  [unwired: 1 in]
            n250 = local write "C settings str"(w317) -> ()
            n251 = local read "Protocol list"() -> (w335:string[])
            n252 = Insert Into Array(array=w335, index=w314, new element=w323) -> (w336:string[])
            n253 = local write "Protocol list"(w336) -> ()
            n254 = Concatenate Strings("C", w330, w320, w330, w318) -> (w319:string)
            n255 = case shown="500" w334 {
              tunnel: w319 -> [w344 w354 w393 w449]
              frame 500 {
                n256 = local read "iteration"() -> (w346:i32)
                n257 = local read "counter"() -> (w350:i32)
                n258 = local read "C settings"() -> (w353:dbl[])
                n259 = local read "Group array settings"() -> (w352:dbl[][])
                n260 = Add(x=w346, y=w350) -> (x+y=w340:i32)
                n261 = Insert Into Array(array=w352, index (col)=w340, new element=w353) -> (w351:dbl[][])  [unwired: 1 in]
                n262 = local write "Group array settings"(w351) -> ()
                n263 = Concatenate Strings(w344, "_01.dat") -> (w345:string)
                n264 = local read "First file array"() -> (w341:bool[])
                n265 = local read "File name"() -> (w349:string[])
                n266 = Insert Into Array(array=w341, index=w340, new element=TRUE) -> (w342:bool[])
                n267 = local write "First file array"(w342) -> ()
                n268 = Insert Into Array(array=w349, index=w340, new element=w345) -> (w348:string[])
                n269 = local write "File name"(w348) -> ()
              }
              frame 1000, Default {
                n270 = local read "C settings"() -> (w360:dbl[])
                n271 = Replace Array Subset(array=w360, new element=500.0 ("new element/subarray"), index=2) -> (w355:dbl[])
                n272 = flat-sequence {
                  tunnel: w355 -> [w372]
                  tunnel: w354 -> [w367]
                  tunnel: [w367] -> w356
                  tunnel: [w375] -> w357
                  tunnel: w356 -> [w375]
                  tunnel: w355 -> [w387]
                  tunnel: w357 -> [w386]
                  frame #0 {
                    n273 = local read "iteration"() -> (w371:i32)
                    n274 = local read "counter"() -> (w370:i32)
                    n275 = Concatenate Strings(w367, "_01.dat") -> (w368:string)
                    n276 = local read "Group array settings"() -> (w373:dbl[][])
                    n277 = Add(x=w371, y=w370) -> (x+y=w361:i32)
                    n278 = local read "First file array"() -> (w362:bool[])
                    n279 = local read "File name"() -> (w366:string[])
                    n280 = Insert Into Array(array=w366, index=w361, new element=w368) -> (w365:string[])
                    n281 = local write "File name"(w365) -> ()
                    n282 = Insert Into Array(array=w362, index=w361, new element=TRUE) -> (w363:bool[])
                    n283 = local write "First file array"(w363) -> ()
                    n284 = Insert Into Array(array=w373, index (col)=w361, new element=w372) -> (w374:dbl[][])  [unwired: 1 in]
                    n285 = local write "Group array settings"(w374) -> ()
                  }
                  frame #1 {
                    n286 = local read "counter"() -> (w377:i32)
                    n287 = Increment(x=w377) -> (x+1=w376:i32)
                    n288 = local write "counter"(w376) -> ()
                  }
                  frame #2 {
                    n289 = local read "iteration"() -> (w388:i32)
                    n290 = local read "counter"() -> (w389:i32)
                    n291 = Concatenate Strings(w386, "_02.dat") -> (w384:string)
                    n292 = local read "Group array settings"() -> (w390:dbl[][])
                    n293 = Add(x=w388, y=w389) -> (x+y=w378:i32)
                    n294 = local read "First file array"() -> (w379:bool[])
                    n295 = local read "File name"() -> (w383:string[])
                    n296 = Insert Into Array(array=w383, index=w378, new element=w384) -> (w382:string[])
                    n297 = local write "File name"(w382) -> ()
                    n298 = Insert Into Array(array=w390, index (col)=w378, new element=w387) -> (w391:dbl[][])  [unwired: 1 in]
                    n299 = local write "Group array settings"(w391) -> ()
                    n300 = Insert Into Array(array=w379, index=w378, new element=FALSE) -> (w380:bool[])
                    n301 = local write "First file array"(w380) -> ()
                  }
                }
              }
              frame 1500 {
                n302 = local read "C settings"() -> (w398:dbl[])
                n303 = Replace Array Subset(array=w398, new element=500.0 ("new element/subarray"), index=2) -> (w392:dbl[])
                n304 = flat-sequence {
                  tunnel: w392 -> [w411]
                  tunnel: w393 -> [w408]
                  tunnel: [w408] -> w394
                  tunnel: [w415] -> w397
                  tunnel: w394 -> [w415]
                  tunnel: w392 -> [w425]
                  tunnel: w397 -> [w429]
                  tunnel: [w429] -> w396
                  tunnel: w396 -> [w432]
                  tunnel: [w432] -> w395
                  tunnel: w392 -> [w445]
                  tunnel: w395 -> [w444]
                  frame #0 {
                    n305 = local read "iteration"() -> (w407:i32)
                    n306 = local read "counter"() -> (w412:i32)
                    n307 = Concatenate Strings(w408, "_01.dat") -> (w409:string)
                    n308 = local read "Group array settings"() -> (w414:dbl[][])
                    n309 = Add(x=w407, y=w412) -> (x+y=w401:i32)
                    n310 = local read "First file array"() -> (w402:bool[])
                    n311 = local read "File name"() -> (w406:string[])
                    n312 = Insert Into Array(array=w414, index (col)=w401, new element=w411) -> (w413:dbl[][])  [unwired: 1 in]
                    n313 = local write "Group array settings"(w413) -> ()
                    n314 = Insert Into Array(array=w406, index=w401, new element=w409) -> (w405:string[])
                    n315 = local write "File name"(w405) -> ()
                    n316 = Insert Into Array(array=w402, index=w401, new element=TRUE) -> (w403:bool[])
                    n317 = local write "First file array"(w403) -> ()
                  }
                  frame #1 {
                    n318 = local read "counter"() -> (w417:i32)
                    n319 = Increment(x=w417) -> (x+1=w416:i32)
                    n320 = local write "counter"(w416) -> ()
                  }
                  frame #2 {
                    n321 = local read "iteration"() -> (w424:i32)
                    n322 = local read "counter"() -> (w426:i32)
                    n323 = Concatenate Strings(w429, "_02.dat") -> (w427:string)
                    n324 = local read "Group array settings"() -> (w430:dbl[][])
                    n325 = Add(x=w424, y=w426) -> (x+y=w418:i32)
                    n326 = local read "First file array"() -> (w419:bool[])
                    n327 = local read "File name"() -> (w423:string[])
                    n328 = Insert Into Array(array=w423, index=w418, new element=w427) -> (w422:string[])
                    n329 = local write "File name"(w422) -> ()
                    n330 = Insert Into Array(array=w430, index (col)=w418, new element=w425) -> (w431:dbl[][])  [unwired: 1 in]
                    n331 = local write "Group array settings"(w431) -> ()
                    n332 = Insert Into Array(array=w419, index=w418, new element=FALSE) -> (w420:bool[])
                    n333 = local write "First file array"(w420) -> ()
                  }
                  frame #3 {
                    n334 = local read "counter"() -> (w433:i32)
                    n335 = Increment(x=w433) -> (x+1=w434:i32)
                    n336 = local write "counter"(w434) -> ()
                  }
                  frame #4 {
                    n337 = local read "iteration"() -> (w441:i32)
                    n338 = local read "counter"() -> (w446:i32)
                    n339 = Concatenate Strings(w444, "_03.dat") -> (w442:string)
                    n340 = local read "Group array settings"() -> (w447:dbl[][])
                    n341 = Add(x=w441, y=w446) -> (x+y=w435:i32)
                    n342 = local read "First file array"() -> (w436:bool[])
                    n343 = local read "File name"() -> (w440:string[])
                    n344 = Insert Into Array(array=w440, index=w435, new element=w442) -> (w439:string[])
                    n345 = local write "File name"(w439) -> ()
                    n346 = Insert Into Array(array=w436, index=w435, new element=FALSE) -> (w437:bool[])
                    n347 = local write "First file array"(w437) -> ()
                    n348 = Insert Into Array(array=w447, index (col)=w435, new element=w445) -> (w448:dbl[][])  [unwired: 1 in]
                    n349 = local write "Group array settings"(w448) -> ()
                  }
                }
              }
              frame 2000 {
                n350 = local read "C settings"() -> (w457:dbl[])
                n351 = Replace Array Subset(array=w457, new element=500.0 ("new element/subarray"), index=2) -> (w450:dbl[])
                n352 = flat-sequence {
                  tunnel: w450 -> [w469]
                  tunnel: w449 -> [w466]
                  tunnel: [w466] -> w455
                  tunnel: [w474] -> w456
                  tunnel: w455 -> [w474]
                  tunnel: w450 -> [w485]
                  tunnel: w456 -> [w484]
                  tunnel: [w484] -> w454
                  tunnel: w454 -> [w493]
                  tunnel: [w493] -> w453
                  tunnel: w450 -> [w499]
                  tunnel: w453 -> [w505]
                  tunnel: [w505] -> w452
                  tunnel: w452 -> [w510]
                  tunnel: [w510] -> w451
                  tunnel: w450 -> [w520]
                  tunnel: w451 -> [w519]
                  frame #0 {
                    n353 = local read "iteration"() -> (w471:i32)
                    n354 = local read "counter"() -> (w470:i32)
                    n355 = Concatenate Strings(w466, "_01.dat") -> (w467:string)
                    n356 = local read "Group array settings"() -> (w473:dbl[][])
                    n357 = Add(x=w471, y=w470) -> (x+y=w460:i32)
                    n358 = local read "First file array"() -> (w461:bool[])
                    n359 = local read "File name"() -> (w465:string[])
                    n360 = Insert Into Array(array=w465, index=w460, new element=w467) -> (w464:string[])
                    n361 = local write "File name"(w464) -> ()
                    n362 = Insert Into Array(array=w473, index (col)=w460, new element=w469) -> (w472:dbl[][])  [unwired: 1 in]
                    n363 = local write "Group array settings"(w472) -> ()
                    n364 = Insert Into Array(array=w461, index=w460, new element=TRUE) -> (w462:bool[])
                    n365 = local write "First file array"(w462) -> ()
                  }
                  frame #1 {
                    n366 = local read "counter"() -> (w476:i32)
                    n367 = Increment(x=w476) -> (x+1=w475:i32)
                    n368 = local write "counter"(w475) -> ()
                  }
                  frame #2 {
                    n369 = local read "iteration"() -> (w483:i32)
                    n370 = local read "counter"() -> (w490:i32)
                    n371 = Concatenate Strings(w484, "_02.dat") -> (w488:string)
                    n372 = local read "Group array settings"() -> (w487:dbl[][])
                    n373 = Add(x=w483, y=w490) -> (x+y=w477:i32)
                    n374 = local read "First file array"() -> (w478:bool[])
                    n375 = local read "File name"() -> (w482:string[])
                    n376 = Insert Into Array(array=w482, index=w477, new element=w488) -> (w481:string[])
                    n377 = local write "File name"(w481) -> ()
                    n378 = Insert Into Array(array=w478, index=w477, new element=FALSE) -> (w479:bool[])
                    n379 = local write "First file array"(w479) -> ()
                    n380 = Insert Into Array(array=w487, index (col)=w477, new element=w485) -> (w486:dbl[][])  [unwired: 1 in]
                    n381 = local write "Group array settings"(w486) -> ()
                  }
                  frame #3 {
                    n382 = local read "counter"() -> (w492:i32)
                    n383 = Increment(x=w492) -> (x+1=w491:i32)
                    n384 = local write "counter"(w491) -> ()
                  }
                  frame #4 {
                    n385 = local read "iteration"() -> (w503:i32)
                    n386 = local read "counter"() -> (w506:i32)
                    n387 = Concatenate Strings(w505, "_03.dat") -> (w504:string)
                    n388 = local read "Group array settings"() -> (w500:dbl[][])
                    n389 = Add(x=w503, y=w506) -> (x+y=w494:i32)
                    n390 = local read "First file array"() -> (w495:bool[])
                    n391 = local read "File name"() -> (w502:string[])
                    n392 = Insert Into Array(array=w502, index=w494, new element=w504) -> (w501:string[])
                    n393 = local write "File name"(w501) -> ()
                    n394 = Insert Into Array(array=w500, index (col)=w494, new element=w499) -> (w498:dbl[][])  [unwired: 1 in]
                    n395 = local write "Group array settings"(w498) -> ()
                    n396 = Insert Into Array(array=w495, index=w494, new element=FALSE) -> (w496:bool[])
                    n397 = local write "First file array"(w496) -> ()
                  }
                  frame #5 {
                    n398 = local read "counter"() -> (w509:i32)
                    n399 = Increment(x=w509) -> (x+1=w508:i32)
                    n400 = local write "counter"(w508) -> ()
                  }
                  frame #6 {
                    n401 = local read "iteration"() -> (w517:i32)
                    n402 = local read "counter"() -> (w522:i32)
                    n403 = Concatenate Strings(w519, "_04.dat") -> (w518:string)
                    n404 = local read "Group array settings"() -> (w524:dbl[][])
                    n405 = Add(x=w517, y=w522) -> (x+y=w511:i32)
                    n406 = local read "First file array"() -> (w512:bool[])
                    n407 = local read "File name"() -> (w516:string[])
                    n408 = Insert Into Array(array=w524, index (col)=w511, new element=w520) -> (w521:dbl[][])  [unwired: 1 in]
                    n409 = local write "Group array settings"(w521) -> ()
                    n410 = Insert Into Array(array=w516, index=w511, new element=w518) -> (w515:string[])
                    n411 = local write "File name"(w515) -> ()
                    n412 = Insert Into Array(array=w512, index=w511, new element=FALSE) -> (w513:bool[])
                    n413 = local write "First file array"(w513) -> ()
                  }
                }
              }
            }
            n414 = local read "Main file name"() -> (w322:string[])
            n415 = Insert Into Array(array=w322, index=w314, new element=w319) -> (w321:string[])
            n416 = local write "Main file name"(w321) -> ()
            n417 = Concatenate Strings(w319, "_expinfo.dat") -> (w328:string)
            n418 = local read "Expinfo name"() -> (w332:string[])
            n419 = Insert Into Array(array=w332, index=w314, new element=w328) -> (w331:string[])
            n420 = local write "Expinfo name"(w331) -> ()
            n421 = Concatenate Strings(w319, "_stim.dat") -> (w326:string)
            n422 = local read "Stim file name"() -> (w325:string[])
            n423 = Insert Into Array(array=w325, index=w314, new element=w326) -> (w324:string[])
            n424 = local write "Stim file name"(w324) -> ()
          }
          frame 3, Default {
            (unwired) ""
          }
          frame 0 {
            w578 = "_"
            n425 = while {
              tunnel: [w776] -> w570
              tunnel: [w812] -> w583
              tunnel: ["# Repetitions"] -> w582
              tunnel: [w774] -> w566
              tunnel: [w775] -> w565
              tunnel: [w795] -> w577
              tunnel: [w773] -> w562
              stop <- "Add Button" stop-if-true
              n426 = Get Date/Time In Seconds() -> (seconds since 1Jan1904=w802:timestamp)
              n427 = Format Date/Time String(time format string (%c)="%d", seconds (now)=w802) -> (date/time string=w803:string)  [unwired: 1 in]
              n428 = Format Date/Time String(time format string (%c)="%m", seconds (now)=w802) -> (date/time string=w804:string)  [unwired: 1 in]
              n429 = Format Date/Time String(time format string (%c)="%y", seconds (now)=w802) -> (date/time string=w805:string)  [unwired: 1 in]
              n430 = Format Date/Time String(time format string (%c)="%H", seconds (now)=w802) -> (date/time string=w806:string)  [unwired: 1 in]
              n431 = Format Date/Time String(time format string (%c)="%M", seconds (now)=w802) -> (date/time string=w807:string)  [unwired: 1 in]
              n432 = Format Date/Time String(time format string (%c)="%S", seconds (now)=w802) -> (date/time string=w808:string)  [unwired: 1 in]
              n433 = Concatenate Strings(w803, w804, w805, "_", w806, w807, w808) -> (w795:string)
              n434 = local write "Date_Time"(w795) -> ()
              n435 = Build Array("Amplitude (dB SPL)", "Frequency (Hz)", "Stimulation freq (stim/sec)", "# Repetitions") -> (w812:dbl[])
              n436 = local write "PT settings"(w812) -> ()
              n437 = Number To Decimal String(number=w812) -> (decimal integer string=w773:string[])  [unwired: 1 in]
              n438 = local read "PT words"() -> (w782:string[])
              n439 = Index Array(array=w782) -> (element #1=w777:string, element #2=w778:string, element #3=w779:string, element #4=w780:string, element #5=w781:string, element #6=w783:string, element #7=w784:string, element #8=w785:string, element #9=w786:string, element #10=w787:string, element #11=w789:string, element #12=w790:string, element #13=w791:string)  [unwired: 13 in]
              n440 = Index Array(array=w773) -> (element #1=w774:string, element #2=w775:string, element #3=w788:string, element #4=w792:string)  [unwired: 4 in]
              n441 = Concatenate Strings(w777, w778, w779, w780, w774, w781, w783, w784, w775, w785, w786, w787, w788, w789, w790, w791, w792) -> (w776:string)
            }
            n442 = local read "iteration"() -> (w561:i32)
            n443 = local read "Protocol array settings"() -> (w587:dbl[][])
            n444 = Insert Into Array(array=w587, index (col)=w561, new element=w583) -> (w586:dbl[][])  [unwired: 1 in]
            n445 = local write "Protocol array settings"(w586) -> ()
            n446 = local read "PT settings str"() -> (w564:string[][])
            n447 = Insert Into Array(array=w564, index (col)=w561, new element=w562) -> (w563:string[][])  [unwired: 1 in]
            n448 = local write "PT settings str"(w563) -> ()
            n449 = local read "Protocol list"() -> (w585:string[])
            n450 = Insert Into Array(array=w585, index=w561, new element=w570) -> (w584:string[])
            n451 = local write "Protocol list"(w584) -> ()
            n452 = Concatenate Strings("PT", w565, w578, w566, w578, w577) -> (w567:string)
            n453 = case shown="500" w582 {
              tunnel: w567 -> [w592 w603 w640 w698]
              frame 500 {
                n454 = local read "PT settings"() -> (w601:dbl[])
                n455 = local read "iteration"() -> (w593:i32)
                n456 = local read "counter"() -> (w598:i32)
                n457 = local read "Group array settings"() -> (w600:dbl[][])
                n458 = Add(x=w593, y=w598) -> (x+y=w591:i32)
                n459 = Insert Into Array(array=w600, index (col)=w591, new element=w601) -> (w599:dbl[][])  [unwired: 1 in]
                n460 = local write "Group array settings"(w599) -> ()
                n461 = Concatenate Strings(w592, "_01.dat") -> (w594:string)
                n462 = local read "First file array"() -> (w590:bool[])
                n463 = local read "File name"() -> (w597:string[])
                n464 = Insert Into Array(array=w597, index=w591, new element=w594) -> (w596:string[])
                n465 = local write "File name"(w596) -> ()
                n466 = Insert Into Array(array=w590, index=w591, new element=TRUE) -> (w589:bool[])
                n467 = local write "First file array"(w589) -> ()
              }
              frame 1000, Default {
                n468 = local read "PT settings"() -> (w608:dbl[])
                n469 = Replace Array Subset(array=w608, new element=500.0 ("new element/subarray"), index=3) -> (w602:dbl[])
                n470 = flat-sequence {
                  tunnel: w602 -> [w620]
                  tunnel: w603 -> [w613]
                  tunnel: [w613] -> w604
                  tunnel: [w623] -> w605
                  tunnel: w604 -> [w623]
                  tunnel: w602 -> [w635]
                  tunnel: w605 -> [w634]
                  frame #0 {
                    n471 = local read "iteration"() -> (w619:i32)
                    n472 = local read "counter"() -> (w618:i32)
                    n473 = Concatenate Strings(w613, "_01.dat") -> (w614:string)
                    n474 = local read "Group array settings"() -> (w621:dbl[][])
                    n475 = Add(x=w619, y=w618) -> (x+y=w609:i32)
                    n476 = local read "First file array"() -> (w610:bool[])
                    n477 = local read "File name"() -> (w616:string[])
                    n478 = Insert Into Array(array=w610, index=w609, new element=TRUE) -> (w611:bool[])
                    n479 = local write "First file array"(w611) -> ()
                    n480 = Insert Into Array(array=w616, index=w609, new element=w614) -> (w615:string[])
                    n481 = local write "File name"(w615) -> ()
                    n482 = Insert Into Array(array=w621, index (col)=w609, new element=w620) -> (w622:dbl[][])  [unwired: 1 in]
                    n483 = local write "Group array settings"(w622) -> ()
                  }
                  frame #1 {
                    n484 = local read "counter"() -> (w625:i32)
                    n485 = Increment(x=w625) -> (x+1=w624:i32)
                    n486 = local write "counter"(w624) -> ()
                  }
                  frame #2 {
                    n487 = local read "iteration"() -> (w636:i32)
                    n488 = local read "counter"() -> (w637:i32)
                    n489 = Concatenate Strings(w634, "_02.dat") -> (w630:string)
                    n490 = local read "Group array settings"() -> (w638:dbl[][])
                    n491 = Add(x=w636, y=w637) -> (x+y=w626:i32)
                    n492 = local read "First file array"() -> (w627:bool[])
                    n493 = local read "File name"() -> (w632:string[])
                    n494 = Insert Into Array(array=w632, index=w626, new element=w630) -> (w631:string[])
                    n495 = local write "File name"(w631) -> ()
                    n496 = Insert Into Array(array=w638, index (col)=w626, new element=w635) -> (w639:dbl[][])  [unwired: 1 in]
                    n497 = local write "Group array settings"(w639) -> ()
                    n498 = Insert Into Array(array=w627, index=w626, new element=FALSE) -> (w628:bool[])
                    n499 = local write "First file array"(w628) -> ()
                  }
                }
              }
              frame 1500 {
                n500 = local read "PT settings"() -> (w646:dbl[])
                n501 = Replace Array Subset(array=w646, new element=500.0 ("new element/subarray"), index=3) -> (w641:dbl[])
                n502 = flat-sequence {
                  tunnel: w641 -> [w658]
                  tunnel: w640 -> [w653]
                  tunnel: [w653] -> w642
                  tunnel: [w663] -> w645
                  tunnel: w642 -> [w663]
                  tunnel: w641 -> [w670]
                  tunnel: w645 -> [w674]
                  tunnel: [w674] -> w644
                  tunnel: w644 -> [w680]
                  tunnel: [w680] -> w643
                  tunnel: w641 -> [w692]
                  tunnel: w643 -> [w691]
                  frame #0 {
                    n503 = local read "iteration"() -> (w660:i32)
                    n504 = local read "counter"() -> (w659:i32)
                    n505 = Concatenate Strings(w653, "_01.dat") -> (w655:string)
                    n506 = local read "Group array settings"() -> (w662:dbl[][])
                    n507 = Add(x=w660, y=w659) -> (x+y=w649:i32)
                    n508 = local read "File name"() -> (w654:string[])
                    n509 = local read "First file array"() -> (w650:bool[])
                    n510 = Insert Into Array(array=w654, index=w649, new element=w655) -> (w657:string[])
                    n511 = local write "File name"(w657) -> ()
                    n512 = Insert Into Array(array=w662, index (col)=w649, new element=w658) -> (w661:dbl[][])  [unwired: 1 in]
                    n513 = local write "Group array settings"(w661) -> ()
                    n514 = Insert Into Array(array=w650, index=w649, new element=TRUE) -> (w651:bool[])
                    n515 = local write "First file array"(w651) -> ()
                  }
                  frame #1 {
                    n516 = local read "counter"() -> (w665:i32)
                    n517 = Increment(x=w665) -> (x+1=w664:i32)
                    n518 = local write "counter"(w664) -> ()
                  }
                  frame #2 {
                    n519 = local read "iteration"() -> (w677:i32)
                    n520 = local read "counter"() -> (w671:i32)
                    n521 = Concatenate Strings(w674, "_02.dat") -> (w672:string)
                    n522 = local read "Group array settings"() -> (w678:dbl[][])
                    n523 = Add(x=w677, y=w671) -> (x+y=w666:i32)
                    n524 = local read "First file array"() -> (w667:bool[])
                    n525 = local read "File name"() -> (w676:string[])
                    n526 = Insert Into Array(array=w678, index (col)=w666, new element=w670) -> (w679:dbl[][])  [unwired: 1 in]
                    n527 = local write "Group array settings"(w679) -> ()
                    n528 = Insert Into Array(array=w667, index=w666, new element=FALSE) -> (w668:bool[])
                    n529 = local write "First file array"(w668) -> ()
                    n530 = Insert Into Array(array=w676, index=w666, new element=w672) -> (w675:string[])
                    n531 = local write "File name"(w675) -> ()
                  }
                  frame #3 {
                    n532 = local read "counter"() -> (w681:i32)
                    n533 = Increment(x=w681) -> (x+1=w682:i32)
                    n534 = local write "counter"(w682) -> ()
                  }
                  frame #4 {
                    n535 = local read "iteration"() -> (w694:i32)
                    n536 = local read "counter"() -> (w693:i32)
                    n537 = Concatenate Strings(w691, "_03.dat") -> (w687:string)
                    n538 = local read "Group array settings"() -> (w695:dbl[][])
                    n539 = Add(x=w694, y=w693) -> (x+y=w683:i32)
                    n540 = local read "First file array"() -> (w684:bool[])
                    n541 = local read "File name"() -> (w690:string[])
                    n542 = Insert Into Array(array=w695, index (col)=w683, new element=w692) -> (w696:dbl[][])  [unwired: 1 in]
                    n543 = local write "Group array settings"(w696) -> ()
                    n544 = Insert Into Array(array=w684, index=w683, new element=FALSE) -> (w685:bool[])
                    n545 = local write "First file array"(w685) -> ()
                    n546 = Insert Into Array(array=w690, index=w683, new element=w687) -> (w689:string[])
                    n547 = local write "File name"(w689) -> ()
                  }
                }
              }
              frame 2000 {
                n548 = local read "PT settings"() -> (w705:dbl[])
                n549 = Replace Array Subset(array=w705, new element=500.0 ("new element/subarray"), index=3) -> (w697:dbl[])
                n550 = flat-sequence {
                  tunnel: w697 -> [w717]
                  tunnel: w698 -> [w712]
                  tunnel: [w712] -> w703
                  tunnel: [w722] -> w704
                  tunnel: w703 -> [w722]
                  tunnel: w697 -> [w730]
                  tunnel: w704 -> [w729]
                  tunnel: [w729] -> w702
                  tunnel: w702 -> [w739]
                  tunnel: [w739] -> w701
                  tunnel: w697 -> [w753]
                  tunnel: w701 -> [w750]
                  tunnel: [w750] -> w700
                  tunnel: w700 -> [w756]
                  tunnel: [w756] -> w699
                  tunnel: w697 -> [w768]
                  tunnel: w699 -> [w767]
                  frame #0 {
                    n551 = local read "iteration"() -> (w719:i32)
                    n552 = local read "counter"() -> (w718:i32)
                    n553 = Concatenate Strings(w712, "_01.dat") -> (w713:string)
                    n554 = local read "Group array settings"() -> (w721:dbl[][])
                    n555 = Add(x=w719, y=w718) -> (x+y=w708:i32)
                    n556 = local read "First file array"() -> (w709:bool[])
                    n557 = local read "File name"() -> (w714:string[])
                    n558 = Insert Into Array(array=w714, index=w708, new element=w713) -> (w715:string[])
                    n559 = local write "File name"(w715) -> ()
                    n560 = Insert Into Array(array=w709, index=w708, new element=TRUE) -> (w710:bool[])
                    n561 = local write "First file array"(w710) -> ()
                    n562 = Insert Into Array(array=w721, index (col)=w708, new element=w717) -> (w720:dbl[][])  [unwired: 1 in]
                    n563 = local write "Group array settings"(w720) -> ()
                  }
                  frame #1 {
                    n564 = local read "counter"() -> (w724:i32)
                    n565 = Increment(x=w724) -> (x+1=w723:i32)
                    n566 = local write "counter"(w723) -> ()
                  }
                  frame #2 {
                    n567 = local read "counter"() -> (w737:i32)
                    n568 = local read "iteration"() -> (w738:i32)
                    n569 = Concatenate Strings(w729, "_02.dat") -> (w733:string)
                    n570 = local read "Group array settings"() -> (w732:dbl[][])
                    n571 = Add(x=w738, y=w737) -> (x+y=w725:i32)
                    n572 = local read "First file array"() -> (w726:bool[])
                    n573 = local read "File name"() -> (w735:string[])
                    n574 = Insert Into Array(array=w735, index=w725, new element=w733) -> (w734:string[])
                    n575 = local write "File name"(w734) -> ()
                    n576 = Insert Into Array(array=w726, index=w725, new element=FALSE) -> (w727:bool[])
                    n577 = local write "First file array"(w727) -> ()
                    n578 = Insert Into Array(array=w732, index (col)=w725, new element=w730) -> (w731:dbl[][])  [unwired: 1 in]
                    n579 = local write "Group array settings"(w731) -> ()
                  }
                  frame #3 {
                    n580 = local read "counter"() -> (w741:i32)
                    n581 = Increment(x=w741) -> (x+1=w740:i32)
                    n582 = local write "counter"(w740) -> ()
                  }
                  frame #4 {
                    n583 = local read "iteration"() -> (w746:i32)
                    n584 = local read "counter"() -> (w751:i32)
                    n585 = Concatenate Strings(w750, "_03.dat") -> (w747:string)
                    n586 = local read "Group array settings"() -> (w755:dbl[][])
                    n587 = Add(x=w746, y=w751) -> (x+y=w742:i32)
                    n588 = local read "First file array"() -> (w743:bool[])
                    n589 = local read "File name"() -> (w749:string[])
                    n590 = Insert Into Array(array=w749, index=w742, new element=w747) -> (w748:string[])
                    n591 = local write "File name"(w748) -> ()
                    n592 = Insert Into Array(array=w755, index (col)=w742, new element=w753) -> (w752:dbl[][])  [unwired: 1 in]
                    n593 = local write "Group array settings"(w752) -> ()
                    n594 = Insert Into Array(array=w743, index=w742, new element=FALSE) -> (w744:bool[])
                    n595 = local write "First file array"(w744) -> ()
                  }
                  frame #5 {
                    n596 = local read "counter"() -> (w757:i32)
                    n597 = Increment(x=w757) -> (x+1=w758:i32)
                    n598 = local write "counter"(w758) -> ()
                  }
                  frame #6 {
                    n599 = local read "iteration"() -> (w763:i32)
                    n600 = local read "counter"() -> (w770:i32)
                    n601 = Concatenate Strings(w767, "_04.dat") -> (w764:string)
                    n602 = local read "Group array settings"() -> (w772:dbl[][])
                    n603 = Add(x=w763, y=w770) -> (x+y=w759:i32)
                    n604 = local read "First file array"() -> (w760:bool[])
                    n605 = local read "File name"() -> (w766:string[])
                    n606 = Insert Into Array(array=w772, index (col)=w759, new element=w768) -> (w769:dbl[][])  [unwired: 1 in]
                    n607 = local write "Group array settings"(w769) -> ()
                    n608 = Insert Into Array(array=w766, index=w759, new element=w764) -> (w765:string[])
                    n609 = local write "File name"(w765) -> ()
                    n610 = Insert Into Array(array=w760, index=w759, new element=FALSE) -> (w761:bool[])
                    n611 = local write "First file array"(w761) -> ()
                  }
                }
              }
            }
            n612 = local read "Main file name"() -> (w569:string[])
            n613 = Insert Into Array(array=w569, index=w561, new element=w567) -> (w568:string[])
            n614 = local write "Main file name"(w568) -> ()
            n615 = Concatenate Strings(w567, "_expinfo.dat") -> (w575:string)
            n616 = local read "Expinfo name"() -> (w580:string[])
            n617 = Insert Into Array(array=w580, index=w561, new element=w575) -> (w581:string[])
            n618 = local write "Expinfo name"(w581) -> ()
            n619 = Concatenate Strings(w567, "_stim.dat") -> (w571:string)
            n620 = local read "Stim file name"() -> (w573:string[])
            n621 = Insert Into Array(array=w573, index=w561, new element=w571) -> (w572:string[])
            n622 = local write "Stim file name"(w572) -> ()
          }
        }
        "Tab Control" <- "Type of stimulus"
        "iteration" <- w66
      }
    }
    frame #2 {
      n623 = while {
        stop <- "Start!" stop-if-true
        n624 = Wait (ms)(milliseconds to wait=u32 100) -> ()  [unwired: 1 out]
      }
    }
    frame #3 {
      n625 = local read "How many tests?"() -> (w817:i32)
      n626 = local read "counter"() -> (w818:i32)
      n627 = Add(x=w817, y=w818) -> (x+y=w816:i32)
      n628 = for {
        N: w816 -> [_]
        i -> [w820]
        stop <- "Stop!" stop-if-true
        n629 = local read "Type of stimulus"() -> (w821:u16)
        n630 = case shown="0" w821 {
          tunnel: w820 -> [_ w831 w997 w1155]
          frame 3, Default {
          }
          frame 0 {
            w860 = 10178 items=["Finite Samples"=10178, "Continuous Samples"=10123, "Hardware Timed Single Point"=12522] ("sample mode")
            w865 = 10178 items=["Finite Samples"=10178, "Continuous Samples"=10123, "Hardware Timed Single Point"=12522] ("sample mode")
            # "Stimulation and Adquisition"
            n631 = local read "Output Channel"() -> (w839:tag)
            n632 = local read "Input Channel"() -> (w869:tag)
            n633 = local read "Group array settings"() -> (w870:dbl[][])
            n634 = call-poly <vilib>:"DAQmx Create Virtual Channel.vi"("physical channels"=w869) -> ("task out"=w867:refnum<k21>, "error out"=w868:errorcluster)  [unwired: 13 in]
            n635 = call-poly <vilib>:"DAQmx Create Virtual Channel.vi"("physical channels"=w839) -> ("task out"=w841:refnum<k21>, "error out"=w840:errorcluster)  [unwired: 13 in]
            n636 = call-poly <vilib>:"DAQmx Trigger.vi"("task/channels in"=w867, "source"=tag "/PXI1Slot6/ao/StartTrigger", "error in"=w868) -> ("task out"=w863:refnum<k21>, "error out"=w864:errorcluster)  [unwired: 11 in]
            n637 = Index Array(array=w870, index (row) #1=0 ("disabled index (row)"), index (col) #1=w831, index (row) #2=1, index (col) #2=w831, index (row) #3=2, index (col) #3=w831, index (row) #4=3, index (col) #4=w831) -> (element #1=w834:dbl, element #2=w833:dbl, element #3=w832:dbl, element #4=w823:dbl)
            n638 = local read "Fs (#S/s)"() -> (w826:dbl)
            n639 = call <userlib>:"Pure Tones.vi"("Amplitude (dB SPL)"=w834, "Frequency (Hz)"=w833, "Stimulation freq (stim/sec)"=w832, "Fs (#S/s)"=w826) -> ("Stimulus Waveform"=w857:waveform(dbl), "Signal duration (#S)"=w824:dbl)  [unwired: 3 out]
            n640 = Multiply(x=w824, y=w823) -> (x*y=w850:dbl)
            n641 = call-poly <vilib>:"DAQmx Timing.vi"("task/channels in"=w841, "sample mode"=w860, "samples per channel"=w850, "rate"=w826, "error in"=w840) -> ("task out"=w858:refnum<k21>, "error out"=w859:errorcluster)  [unwired: 9 in]
            n642 = call-poly <vilib>:"DAQmx Timing.vi"("task/channels in"=w863, "sample mode"=w865, "samples per channel"=w850, "rate"=w826, "error in"=w864) -> ("task out"=w861:refnum<k21>, "error out"=w862:errorcluster)  [unwired: 9 in]
            n643 = call <vilib>:"DAQmx Start Task.vi"("task/channels in"=w861, "error in"=w862) -> ("task out"=w851:refnum<k21>, "error out"=w855:errorcluster)  [unwired: 12 in]
            n644 = local write "Stimulus Graph"(w857) -> ()
            n645 = call-poly <vilib>:"DAQmx Write.vi"("task/channels in"=w858, "data"=w857, "error in"=w859) -> ("task out"=w853:refnum<k21>, "error out"=w856:errorcluster)  [unwired: 10 in, 1 out]
            n646 = Merge Errors(w855, w856) -> (w854:errorcluster)
            n647 = call <vilib>:"DAQmx Start Task.vi"("task/channels in"=w853, "error in"=w854) -> ("task out"=w848:refnum<k21>, "error out"=w852:errorcluster)  [unwired: 12 in]
            n648 = call-poly <vilib>:"DAQmx Read.vi"("task/channels in"=w851, "number of samples per channel"=w850, "timeout"=-1.0, "error in"=w852) -> ("task out"=w844:refnum<k21>, "data"=w825:waveform(dbl), "error out"=w847:errorcluster)  [unwired: 9 in]
            n649 = Unbundle By Name(w825) -> ("Y"=w827:dbl[])
            n650 = local write "Acquisition Graph"(w825) -> ()
            n651 = call <vilib>:"DAQmx Is Task Done.vi"("task/channels in"=w848, "error in"=w847) -> ("task out"=w846:refnum<k21>, "task done?"=w836:bool, "error out"=w845:errorcluster)  [unwired: 11 in]
            n652 = Reshape Array(w827, w823, w824) -> (w828:dbl[][])
            n653 = call <vilib>:"DAQmx Clear Task.vi"("task in"=w846, "error in"=w845) -> ("error out"=w843:errorcluster)  [unwired: 13 in]
            n654 = for {
              N: w824 -> [_]
              tunnel: w828 -> [w878]
              tunnel: w823 -> [w875]
              tunnel: [w880] -> w829 mode=indexing
              i -> [w877]
              n655 = Index Array(array=w878, index (col)=w877) -> (element=w876:dbl[])  [unwired: 1 in]
              n656 = Decrement(x=w875) -> (x-1=w879:dbl)
              n657 = while {
                tunnel: w876 -> [w888] mode=indexing
                shift-right: [w886] -> w881
                shift-left: 0.0 -> [w887]
                tunnel: w879 -> [w884]
                i -> [w883]
                stop <- w885 stop-if-true
                n658 = Add(x=w887, y=w888) -> (x+y=w886:dbl)
                n659 = Equal?(x=w883, y=w884) -> (x = y?=w885:bool)
              }
              n660 = Divide(x=w881, y=w875) -> (x/y=w880:dbl)
            }
            n661 = call <vilib>:"DAQmx Clear Task.vi"("task in"=w844, "error in"=w843) -> ("error out"=w842:errorcluster)  [unwired: 13 in]
            n662 = call <vilib>:"Simple Error Handler.vi"("error in (no error)"=w842) -> ()  [unwired: 4 in, 5 out]
            n663 = case shown="True" w836 {
              tunnel: [_ w985] -> w838
              tunnel: w831 -> [_ w980]
              tunnel: w825 -> [_ w979]
              frame False {
              }
              frame True {
                n664 = local read "File name"() -> (w987:string[])
                n665 = Unbundle By Name(w979) -> ("Y"=w978:dbl[])
                n666 = local read "File path"() -> (w981:path)
                n667 = Array To Spreadsheet String(array=w978, 3:"%f" ("text")) -> (spreadsheet string=w983:string)  [unwired: 1 in]
                n668 = Index Array(array=w987, index=w980) -> (element=w982:string)
                n669 = Build Path(base path=w981, name or relative path=w982) -> (appended path=w986:path)
                n670 = Write to Text File(file (use dialog)=w986, text=w983) -> (error out=w985:errorcluster)  [unwired: 2 in, 2 out]
              }
            }
            n671 = Reciprocal(x=w826) -> (1/x=w830:dbl)
            n672 = Bundle By Name("Y"=w829, "dt"=w830) -> (w822:waveform(dbl))  [unwired: 1 in]
            n673 = local read "First file array"() -> (w837:bool[])
            n674 = local write "Averaged Acq Graph"(w822) -> ()
            n675 = Index Array(array=w837, index=w831) -> (element=w835:bool)
            n676 = call <vilib>:"Simple Error Handler.vi"("error in (no error)"=w838) -> ()  [unwired: 4 in, 5 out]
            n677 = case shown="True" w835 {
              tunnel: w834 -> [_ w967]
              tunnel: w833 -> [_ w966]
              tunnel: w832 -> [_ w965]
              tunnel: w826 -> [_ w964]
              tunnel: w831 -> [_ w962]
              frame False {
                n678 = local read "counter 2"() -> (w890:i32)
                n679 = Increment(x=w890) -> (x+1=w889:i32)
                n680 = local write "counter 2"(w889) -> ()
              }
              frame True {
                # "Saving experiment information"
                # "Saving stimulus information"
                n681 = local read "counter 2"() -> (w963:i32)
                n682 = Multiply(x=10.0, y=w967) -> (x*y=w968:dbl)
                n683 = call <userlib>:"Pure Tones.vi"("Amplitude (dB SPL)"=w968, "Frequency (Hz)"=w966, "Stimulation freq (stim/sec)"=w965, "Fs (#S/s)"=w964) -> ("Signal duration (ms)"=w933:dbl, "Stimulus Waveform"=w970:waveform(dbl), "Stimulus duration (ms)"=w932:dbl, "Delay (ms)"=w931:dbl)  [unwired: 1 out]
                n684 = Subtract(x=w962, y=w963) -> (x-y=w891:i32)
                n685 = local read "Stim file name"() -> (w974:string[])
                n686 = Unbundle By Name(w970) -> ("Y"=w976:dbl[])
                n687 = Array To Spreadsheet String(array=w976, 3:"%f" ("text")) -> (spreadsheet string=w971:string)  [unwired: 1 in]
                n688 = local read "File path"() -> (w973:path)
                n689 = Index Array(array=w974, index=w891) -> (element=w972:string)
                n690 = local read "Expinfo words"() -> (w956:string[])
                n691 = Build Path(base path=w973, name or relative path=w972) -> (appended path=w975:path)
                n692 = Write to Text File(file (use dialog)=w975, text=w971) -> (error out=w929:errorcluster)  [unwired: 2 in, 2 out]
                n693 = Index Array(array=w956) -> (element #1=w955:string, element #2=w954:string, element #3=w952:string, element #4=w951:string, element #5=w950:string, element #6=w948:string, element #7=w947:string, element #8=w946:string, element #9=w944:string, element #10=w943:string, element #11=w942:string, element #12=w940:string, element #13=w939:string, element #14=w938:string, element #15=w936:string, element #16=w935:string, element #17=w934:string, element #18=w904:string, element #19=w903:string, element #20=w902:string, element #21=w900:string, element #22=w899:string, element #23=w898:string, element #24=w896:string, element #25=w895:string, element #26=w894:string)  [unwired: 26 in]
                n694 = local read "Main file name"() -> (w957:string[])
                n695 = local read "PT settings str"() -> (w922:string[][])
                n696 = local read "PT words"() -> (w928:string[])
                n697 = local read "User name"() -> (w953:string)
                n698 = local read "Subject ID"() -> (w949:string)
                n699 = local read "File path str"() -> (w941:string)
                n700 = local read "Fs"() -> (w937:string)
                n701 = Index Array(array=w922, index (row) #1=0 ("disabled index (row)"), index (col) #1=w891, index (row) #2=1 ("disabled index (row)"), index (col) #2=w891, index (row) #3=2 ("disabled index (row)"), index (col) #3=w891, index (row) #4=3 ("disabled index (row)"), index (col) #4=w891) -> (element #1=w921:string, element #2=w913:string, element #3=w909:string, element #4=w905:string)
                n702 = Index Array(array=w957, index=w891) -> (element=w945:string)
                n703 = Index Array(array=w928) -> (element #1=w927:string, element #2=w926:string, element #3=w925:string, element #4=w924:string, element #5=w916:string, element #6=w915:string, element #7=w914:string, element #8=w912:string, element #9=w911:string, element #10=w910:string, element #11=w908:string, element #12=w907:string, element #13=w906:string)  [unwired: 14 in, 1 out]
                n704 = Number To Decimal String(number=w933) -> (decimal integer string=w901:string)  [unwired: 1 in]
                n705 = Number To Decimal String(number=w932) -> (decimal integer string=w897:string)  [unwired: 1 in]
                n706 = Number To Decimal String(number=w931) -> (decimal integer string=w893:string)  [unwired: 1 in]
                n707 = Concatenate Strings(w955, w954, w953, w952, w951, w950, w949, w948, w947, w946, w945, w944, w943, w942, w941, w940, w939, w938, w937, w936, w935, w934, w927, w926, w925, w924, w921, w916, w915, w914, w913, w912, w911, w910, w909, w908, w907, w906, w905, w904, w903, w902, w901, w900, w899, w898, w897, w896, w895, w894, w893) -> (w930:string)
                n708 = local read "Expinfo name"() -> (w960:string[])
                n709 = Increment(x=w891) -> (x+1=w892:i32)
                n710 = local write "Current test"(w892) -> ()
                n711 = local read "File path"() -> (w959:path)
                n712 = Index Array(array=w960, index=w891) -> (element=w961:string)
                n713 = Build Path(base path=w959, name or relative path=w961) -> (appended path=w923:path)
                n714 = Write to Text File(file (use dialog)=w923, text=w930, error in=w929) -> (error out=w958:errorcluster)  [unwired: 1 in, 2 out]
                n715 = call <vilib>:"Simple Error Handler.vi"("error in (no error)"=w958) -> ()  [unwired: 4 in, 5 out]
              }
            }
          }
          frame 1 {
            w1024 = 10178 items=["Finite Samples"=10178, "Continuous Samples"=10123, "Hardware Timed Single Point"=12522] ("sample mode")
            w1030 = 10178 items=["Finite Samples"=10178, "Continuous Samples"=10123, "Hardware Timed Single Point"=12522] ("sample mode")
            # "Stimulation and Adquisition"
            n716 = local read "Output Channel"() -> (w1025:tag)
            n717 = local read "Input Channel"() -> (w1034:tag)
            n718 = local read "Group array settings"() -> (w1038:dbl[][])
            n719 = call-poly <vilib>:"DAQmx Create Virtual Channel.vi"("physical channels"=w1034) -> ("task out"=w1032:refnum<k21>, "error out"=w1033:errorcluster)  [unwired: 13 in]
            n720 = call-poly <vilib>:"DAQmx Create Virtual Channel.vi"("physical channels"=w1025) -> ("task out"=w1006:refnum<k21>, "error out"=w1007:errorcluster)  [unwired: 13 in]
            n721 = call-poly <vilib>:"DAQmx Trigger.vi"("task/channels in"=w1032, "source"=tag "/PXI1Slot6/ao/StartTrigger", "error in"=w1033) -> ("task out"=w1028:refnum<k21>, "error out"=w1029:errorcluster)  [unwired: 11 in]
            n722 = local read "Fs (#S/s)"() -> (w991:dbl)
            n723 = Index Array(array=w1038, index (row) #1=0 ("disabled index (row)"), index (col) #1=w997, index (row) #2=1, index (col) #2=w997, index (row) #3=2, index (col) #3=w997) -> (element #1=w999:dbl, element #2=w998:dbl, element #3=w988:dbl)
            n724 = call <userlib>:"White Noise.vi"("Amplitude (dB SPL)"=w999, "Stimulation freq (stim/sec)"=w998, "Fs (#S/s)"=w991) -> ("Stimulus Waveform"=w1005:waveform(dbl), "Signal duration (#S)"=w989:dbl)  [unwired: 3 out]
            n725 = Multiply(x=w989, y=w988) -> (x*y=w1004:dbl)
            n726 = call-poly <vilib>:"DAQmx Timing.vi"("task/channels in"=w1006, "sample mode"=w1024, "samples per channel"=w1004, "rate"=w991, "error in"=w1007) -> ("task out"=w1022:refnum<k21>, "error out"=w1023:errorcluster)  [unwired: 9 in]
            n727 = call-poly <vilib>:"DAQmx Timing.vi"("task/channels in"=w1028, "sample mode"=w1030, "samples per channel"=w1004, "rate"=w991, "error in"=w1029) -> ("task out"=w1026:refnum<k21>, "error out"=w1027:errorcluster)  [unwired: 9 in]
            n728 = call <vilib>:"DAQmx Start Task.vi"("task/channels in"=w1026, "error in"=w1027) -> ("task out"=w1016:refnum<k21>, "error out"=w1020:errorcluster)  [unwired: 12 in]
            n729 = local write "Stimulus Graph"(w1005) -> ()
            n730 = call-poly <vilib>:"DAQmx Write.vi"("task/channels in"=w1022, "data"=w1005, "error in"=w1023) -> ("task out"=w1018:refnum<k21>, "error out"=w1021:errorcluster)  [unwired: 10 in, 1 out]
            n731 = Merge Errors(w1020, w1021) -> (w1019:errorcluster)
            n732 = call <vilib>:"DAQmx Start Task.vi"("task/channels in"=w1018, "error in"=w1019) -> ("task out"=w1014:refnum<k21>, "error out"=w1017:errorcluster)  [unwired: 12 in]
            n733 = call-poly <vilib>:"DAQmx Read.vi"("task/channels in"=w1016, "number of samples per channel"=w1004, "timeout"=-1.0, "error in"=w1017) -> ("task out"=w1010:refnum<k21>, "data"=w990:waveform(dbl), "error out"=w1013:errorcluster)  [unwired: 9 in]
            n734 = local write "Acquisition Graph"(w990) -> ()
            n735 = call <vilib>:"DAQmx Is Task Done.vi"("task/channels in"=w1014, "error in"=w1013) -> ("task out"=w1012:refnum<k21>, "task done?"=w1003:bool, "error out"=w1011:errorcluster)  [unwired: 11 in]
            n736 = Unbundle By Name(w990) -> ("Y"=w993:dbl[])
            n737 = call <vilib>:"DAQmx Clear Task.vi"("task in"=w1012, "error in"=w1011) -> ("error out"=w1009:errorcluster)  [unwired: 13 in]
            n738 = Reshape Array(w993, w988, w989) -> (w994:dbl[][])
            n739 = for {
              N: w989 -> [_]
              tunnel: w994 -> [w1042]
              tunnel: w988 -> [w1039]
              tunnel: [w1044] -> w995 mode=indexing
              i -> [w1041]
              n740 = Index Array(array=w1042, index (col)=w1041) -> (element=w1040:dbl[])  [unwired: 1 in]
              n741 = Decrement(x=w1039) -> (x-1=w1043:dbl)
              n742 = while {
                tunnel: w1040 -> [w1052] mode=indexing
                shift-right: [w1050] -> w1045
                shift-left: 0.0 -> [w1051]
                tunnel: w1043 -> [w1048]
                i -> [w1047]
                stop <- w1049 stop-if-true
                n743 = Add(x=w1051, y=w1052) -> (x+y=w1050:dbl)
                n744 = Equal?(x=w1047, y=w1048) -> (x = y?=w1049:bool)
              }
              n745 = Divide(x=w1045, y=w1039) -> (x/y=w1044:dbl)
            }
            n746 = call <vilib>:"DAQmx Clear Task.vi"("task in"=w1010, "error in"=w1009) -> ("error out"=w1008:errorcluster)  [unwired: 13 in]
            n747 = call <vilib>:"Simple Error Handler.vi"("error in (no error)"=w1008) -> ()  [unwired: 4 in, 5 out]
            n748 = case shown="True" w1003 {
              tunnel: [_ w1137] -> w1002
              tunnel: w990 -> [_ w1140]
              tunnel: w997 -> [_ w1136]
              frame False {
              }
              frame True {
                n749 = Unbundle By Name(w1140) -> ("Y"=w1139:dbl[])
                n750 = local read "File name"() -> (w1144:string[])
                n751 = local read "File path"() -> (w1145:path)
                n752 = Array To Spreadsheet String(array=w1139, 3:"%f" ("text")) -> (spreadsheet string=w1141:string)  [unwired: 1 in]
                n753 = Index Array(array=w1144, index=w1136) -> (element=w1143:string)
                n754 = Build Path(base path=w1145, name or relative path=w1143) -> (appended path=w1138:path)
                n755 = Write to Text File(file (use dialog)=w1138, text=w1141) -> (error out=w1137:errorcluster)  [unwired: 2 in, 2 out]
              }
            }
            n756 = Reciprocal(x=w991) -> (1/x=w996:dbl)
            n757 = Bundle By Name("Y"=w995, "dt"=w996) -> (w992:waveform(dbl))  [unwired: 1 in]
            n758 = local read "First file array"() -> (w1000:bool[])
            n759 = local write "Averaged Acq Graph"(w992) -> ()
            n760 = call <vilib>:"Simple Error Handler.vi"("error in (no error)"=w1002) -> ()  [unwired: 4 in, 5 out]
            n761 = Index Array(array=w1000, index=w997) -> (element=w1001:bool)
            n762 = case shown="True" w1001 {
              tunnel: w999 -> [_ w1133]
              tunnel: w998 -> [_ w1132]
              tunnel: w991 -> [_ w1131]
              tunnel: w997 -> [_ w1129]
              frame False {
                n763 = local read "counter 2"() -> (w1054:i32)
                n764 = Increment(x=w1054) -> (x+1=w1053:i32)
                n765 = local write "counter 2"(w1053) -> ()
              }
              frame True {
                # "Saving experiment information"
                # "Saving stimulus information"
                n766 = local read "counter 2"() -> (w1130:i32)
                n767 = Multiply(x=10.0, y=w1133) -> (x*y=w1135:dbl)
                n768 = call <userlib>:"White Noise.vi"("Amplitude (dB SPL)"=w1135, "Stimulation freq (stim/sec)"=w1132, "Fs (#S/s)"=w1131) -> ("Stimulus Waveform"=w1121:waveform(dbl), "Stimulus duration (ms)"=w1095:dbl, "Delay (ms)"=w1094:dbl, "Signal duration (ms)"=w1096:dbl)  [unwired: 1 out]
                n769 = Subtract(x=w1129, y=w1130) -> (x-y=w1055:i32)
                n770 = local read "Stim file name"() -> (w1122:string[])
                n771 = Unbundle By Name(w1121) -> ("Y"=w1127:dbl[])
                n772 = Array To Spreadsheet String(array=w1127, 3:"%f" ("text")) -> (spreadsheet string=w1128:string)  [unwired: 1 in]
                n773 = local read "File path"() -> (w1123:path)
                n774 = Index Array(array=w1122, index=w1055) -> (element=w1125:string)
                n775 = Build Path(base path=w1123, name or relative path=w1125) -> (appended path=w1124:path)
                n776 = local read "Expinfo words"() -> (w1103:string[])
                n777 = Write to Text File(file (use dialog)=w1124, text=w1128) -> (error out=w1088:errorcluster)  [unwired: 2 in, 2 out]
                n778 = Index Array(array=w1103) -> (element #1=w1104:string, element #2=w1105:string, element #3=w1106:string, element #4=w1107:string, element #5=w1108:string, element #6=w1109:string, element #7=w1110:string, element #8=w1111:string, element #9=w1112:string, element #10=w1113:string, element #11=w1114:string, element #12=w1115:string, element #13=w1116:string, element #14=w1117:string, element #15=w1118:string, element #16=w1119:string, element #17=w1120:string, element #18=w1068:string, element #19=w1067:string, element #20=w1066:string, element #21=w1064:string, element #22=w1063:string, element #23=w1062:string, element #24=w1060:string, element #25=w1059:string, element #26=w1058:string)  [unwired: 26 in]
                n779 = local read "Main file name"() -> (w1101:string[])
                n780 = local read "WN words"() -> (w1087:string[])
                n781 = local read "WN settings str"() -> (w1086:string[][])
                n782 = local read "File path str"() -> (w1098:string)
                n783 = local read "User name"() -> (w1102:string)
                n784 = local read "Subject ID"() -> (w1100:string)
                n785 = local read "Fs"() -> (w1097:string)
                n786 = Index Array(array=w1101, index=w1055) -> (element=w1099:string)
                n787 = Index Array(array=w1087) -> (element #1=w1082:string, element #2=w1081:string, element #3=w1080:string, element #4=w1079:string, element #5=w1076:string, element #6=w1075:string, element #7=w1074:string, element #8=w1072:string, element #9=w1071:string, element #10=w1070:string)  [unwired: 10 in]
                n788 = Index Array(array=w1086, index (row) #1=0 ("disabled index (row)"), index (col) #1=w1055, index (row) #2=1 ("disabled index (row)"), index (col) #2=w1055, index (row) #3=2 ("disabled index (row)"), index (col) #3=w1055) -> (element #1=w1078:string, element #2=w1073:string, element #3=w1069:string)
                n789 = Number To Decimal String(number=w1096) -> (decimal integer string=w1065:string)  [unwired: 1 in]
                n790 = Number To Decimal String(number=w1095) -> (decimal integer string=w1061:string)  [unwired: 1 in]
                n791 = Number To Decimal String(number=w1094) -> (decimal integer string=w1057:string)  [unwired: 1 in]
                n792 = Concatenate Strings(w1104, w1105, w1102, w1106, w1107, w1108, w1100, w1109, w1110, w1111, w1099, w1112, w1113, w1114, w1098, w1115, w1116, w1117, w1097, w1118, w1119, w1120, w1082, w1081, w1080, w1079, w1078, w1076, w1075, w1074, w1073, w1072, w1071, w1070, w1069, w1068, w1067, w1066, w1065, w1064, w1063, w1062, w1061, w1060, w1059, w1058, w1057) -> (w1091:string)
                n793 = local read "Expinfo name"() -> (w1090:string[])
                n794 = Increment(x=w1055) -> (x+1=w1056:i32)
                n795 = local write "Current test"(w1056) -> ()
                n796 = local read "File path"() -> (w1089:path)
                n797 = Index Array(array=w1090, index=w1055) -> (element=w1092:string)
                n798 = Build Path(base path=w1089, name or relative path=w1092) -> (appended path=w1077:path)
                n799 = Write to Text File(file (use dialog)=w1077, text=w1091, error in=w1088) -> (error out=w1093:errorcluster)  [unwired: 1 in, 2 out]
                n800 = call <vilib>:"Simple Error Handler.vi"("error in (no error)"=w1093) -> ()  [unwired: 4 in, 5 out]
              }
            }
          }
          frame 2 {
            w1174 = 10178 items=["Finite Samples"=10178, "Continuous Samples"=10123, "Hardware Timed Single Point"=12522] ("sample mode")
            w1168 = 10178 items=["Finite Samples"=10178, "Continuous Samples"=10123, "Hardware Timed Single Point"=12522] ("sample mode")
            # "Stimulation and Adquisition"
            n801 = local read "Input Channel"() -> (w1164:tag)
            n802 = local read "Output Channel"() -> (w1173:tag)
            n803 = local read "Group array settings"() -> (w1196:dbl[][])
            n804 = call-poly <vilib>:"DAQmx Create Virtual Channel.vi"("physical channels"=w1164) -> ("task out"=w1166:refnum<k21>, "error out"=w1165:errorcluster)  [unwired: 13 in]
            n805 = call-poly <vilib>:"DAQmx Create Virtual Channel.vi"("physical channels"=w1173) -> ("task out"=w1192:refnum<k21>, "error out"=w1191:errorcluster)  [unwired: 13 in]
            n806 = local read "Fs (#S/s)"() -> (w1147:dbl)
            n807 = call-poly <vilib>:"DAQmx Trigger.vi"("task/channels in"=w1166, "source"=tag "/PXI1Slot6/ao/StartTrigger", "error in"=w1165) -> ("task out"=w1170:refnum<k21>, "error out"=w1169:errorcluster)  [unwired: 11 in]
            n808 = Index Array(array=w1196, index (row) #1=0 ("disabled index (row)"), index (col) #1=w1155, index (row) #2=1, index (col) #2=w1155, index (row) #3=2, index (col) #3=w1155) -> (element #1=w1157:dbl, element #2=w1156:dbl, element #3=w1148:dbl)
            n809 = call <userlib>:"Clic.vi"("Amplitude (dB SPL)"=w1157, "Stimulation freq (stim/sec)"=w1156, "Fs (#S/s)"=w1147) -> ("Stimulus Waveform"=w1163:waveform(dbl), "Signal duration (#S)"=w1149:dbl)  [unwired: 3 out]
            n810 = Multiply(x=w1149, y=w1148) -> (x*y=w1161:dbl)
            n811 = call-poly <vilib>:"DAQmx Timing.vi"("task/channels in"=w1192, "sample mode"=w1174, "samples per channel"=w1161, "rate"=w1147, "error in"=w1191) -> ("task out"=w1176:refnum<k21>, "error out"=w1175:errorcluster)  [unwired: 9 in]
            n812 = call-poly <vilib>:"DAQmx Timing.vi"("task/channels in"=w1170, "sample mode"=w1168, "samples per channel"=w1161, "rate"=w1147, "error in"=w1169) -> ("task out"=w1172:refnum<k21>, "error out"=w1171:errorcluster)  [unwired: 9 in]
            n813 = call <vilib>:"DAQmx Start Task.vi"("task/channels in"=w1172, "error in"=w1171) -> ("task out"=w1182:refnum<k21>, "error out"=w1178:errorcluster)  [unwired: 12 in]
            n814 = local write "Stimulus Graph"(w1163) -> ()
            n815 = call-poly <vilib>:"DAQmx Write.vi"("task/channels in"=w1176, "data"=w1163, "error in"=w1175) -> ("task out"=w1180:refnum<k21>, "error out"=w1177:errorcluster)  [unwired: 10 in, 1 out]
            n816 = Merge Errors(w1178, w1177) -> (w1179:errorcluster)
            n817 = call <vilib>:"DAQmx Start Task.vi"("task/channels in"=w1180, "error in"=w1179) -> ("task out"=w1184:refnum<k21>, "error out"=w1181:errorcluster)  [unwired: 12 in]
            n818 = call-poly <vilib>:"DAQmx Read.vi"("task/channels in"=w1182, "number of samples per channel"=w1161, "timeout"=-1.0, "error in"=w1181) -> ("task out"=w1188:refnum<k21>, "data"=w1150:waveform(dbl), "error out"=w1185:errorcluster)  [unwired: 9 in]
            n819 = Unbundle By Name(w1150) -> ("Y"=w1151:dbl[])
            n820 = call <vilib>:"DAQmx Is Task Done.vi"("task/channels in"=w1184, "error in"=w1185) -> ("task out"=w1186:refnum<k21>, "task done?"=w1162:bool, "error out"=w1187:errorcluster)  [unwired: 11 in]
            n821 = local write "Acquisition Graph"(w1150) -> ()
            n822 = Reshape Array(w1151, w1148, w1149) -> (w1152:dbl[][])
            n823 = call <vilib>:"DAQmx Clear Task.vi"("task in"=w1186, "error in"=w1187) -> ("error out"=w1189:errorcluster)  [unwired: 13 in]
            n824 = for {
              N: w1149 -> [_]
              tunnel: w1152 -> [w1200]
              tunnel: w1148 -> [w1197]
              tunnel: [w1202] -> w1153 mode=indexing
              i -> [w1199]
              n825 = Index Array(array=w1200, index (col)=w1199) -> (element=w1198:dbl[])  [unwired: 1 in]
              n826 = Decrement(x=w1197) -> (x-1=w1201:dbl)
              n827 = while {
                tunnel: w1198 -> [w1210] mode=indexing
                shift-right: [w1208] -> w1203
                shift-left: 0.0 -> [w1209]
                tunnel: w1201 -> [w1206]
                i -> [w1205]
                stop <- w1207 stop-if-true
                n828 = Add(x=w1209, y=w1210) -> (x+y=w1208:dbl)
                n829 = Equal?(x=w1205, y=w1206) -> (x = y?=w1207:bool)
              }
              n830 = Divide(x=w1203, y=w1197) -> (x/y=w1202:dbl)
            }
            n831 = call <vilib>:"DAQmx Clear Task.vi"("task in"=w1188, "error in"=w1189) -> ("error out"=w1190:errorcluster)  [unwired: 13 in]
            n832 = call <vilib>:"Simple Error Handler.vi"("error in (no error)"=w1190) -> ()  [unwired: 4 in, 5 out]
            n833 = case shown="True" w1162 {
              tunnel: w1150 -> [_ w1298]
              tunnel: [_ w1296] -> w1160
              tunnel: w1155 -> [_ w1295]
              frame False {
              }
              frame True {
                n834 = Unbundle By Name(w1298) -> ("Y"=w1297:dbl[])
                n835 = local read "File name"() -> (w1300:string[])
                n836 = local read "File path"() -> (w1303:path)
                n837 = Index Array(array=w1300, index=w1295) -> (element=w1299:string)
                n838 = Array To Spreadsheet String(array=w1297, 3:"%f" ("text")) -> (spreadsheet string=w1301:string)  [unwired: 1 in]
                n839 = Build Path(base path=w1303, name or relative path=w1299) -> (appended path=w1294:path)
                n840 = Write to Text File(file (use dialog)=w1294, text=w1301) -> (error out=w1296:errorcluster)  [unwired: 2 in, 2 out]
              }
            }
            n841 = Reciprocal(x=w1147) -> (1/x=w1154:dbl)
            n842 = Bundle By Name("Y"=w1153, "dt"=w1154) -> (w1146:waveform(dbl))  [unwired: 1 in]
            n843 = local read "First file array"() -> (w1158:bool[])
            n844 = local write "Averaged Acq Graph"(w1146) -> ()
            n845 = call <vilib>:"Simple Error Handler.vi"("error in (no error)"=w1160) -> ()  [unwired: 4 in, 5 out]
            n846 = Index Array(array=w1158, index=w1155) -> (element=w1159:bool)
            n847 = case shown="True" w1159 {
              tunnel: w1157 -> [_ w1291]
              tunnel: w1156 -> [_ w1290]
              tunnel: w1147 -> [_ w1289]
              tunnel: w1155 -> [_ w1287]
              frame False {
                n848 = local read "counter 2"() -> (w1212:i32)
                n849 = Increment(x=w1212) -> (x+1=w1211:i32)
                n850 = local write "counter 2"(w1211) -> ()
              }
              frame True {
                # "Saving experiment information"
                # "Saving stimulus information"
                n851 = local read "counter 2"() -> (w1288:i32)
                n852 = Multiply(x=10.0, y=w1291) -> (x*y=w1293:dbl)
                n853 = call <userlib>:"Clic.vi"("Amplitude (dB SPL)"=w1293, "Stimulation freq (stim/sec)"=w1290, "Fs (#S/s)"=w1289) -> ("Stimulus Waveform"=w1280:waveform(dbl), "Stimulus duration (ms)"=w1276:dbl, "Delay (ms)"=w1275:dbl, "Signal duration (ms)"=w1277:dbl)  [unwired: 1 out]
                n854 = Subtract(x=w1287, y=w1288) -> (x-y=w1213:i32)
                n855 = local read "Stim file name"() -> (w1286:string[])
                n856 = Unbundle By Name(w1280) -> ("Y"=w1282:dbl[])
                n857 = Array To Spreadsheet String(array=w1282, 3:"%f" ("text")) -> (spreadsheet string=w1283:string)  [unwired: 1 in]
                n858 = local read "File path"() -> (w1284:path)
                n859 = Index Array(array=w1286, index=w1213) -> (element=w1285:string)
                n860 = Build Path(base path=w1284, name or relative path=w1285) -> (appended path=w1279:path)
                n861 = local read "Expinfo words"() -> (w1242:string[])
                n862 = Write to Text File(file (use dialog)=w1279, text=w1283) -> (error out=w1270:errorcluster)  [unwired: 2 in, 2 out]
                n863 = local read "Main file name"() -> (w1278:string[])
                n864 = Index Array(array=w1242) -> (element #1=w1252:string, element #2=w1253:string, element #3=w1254:string, element #4=w1255:string, element #5=w1256:string, element #6=w1257:string, element #7=w1258:string, element #8=w1259:string, element #9=w1260:string, element #10=w1261:string, element #11=w1262:string, element #12=w1263:string, element #13=w1264:string, element #14=w1265:string, element #15=w1266:string, element #16=w1267:string, element #17=w1268:string, element #18=w1251:string, element #19=w1250:string, element #20=w1249:string, element #21=w1248:string, element #22=w1247:string, element #23=w1246:string, element #24=w1245:string, element #25=w1244:string, element #26=w1243:string)  [unwired: 26 in]
                n865 = local read "C settings str"() -> (w1237:string[][])
                n866 = local read "C words"() -> (w1238:string[])
                n867 = local read "File path str"() -> (w1233:string)
                n868 = local read "User name"() -> (w1236:string)
                n869 = local read "Subject ID"() -> (w1235:string)
                n870 = local read "Fs"() -> (w1232:string)
                n871 = Index Array(array=w1278, index=w1213) -> (element=w1234:string)
                n872 = Index Array(array=w1237, index (row) #1=0 ("disabled index (row)"), index (col) #1=w1213, index (row) #2=1 ("disabled index (row)"), index (col) #2=w1213, index (row) #3=2 ("disabled index (row)"), index (col) #3=w1213) -> (element #1=w1227:string, element #2=w1223:string, element #3=w1219:string)
                n873 = Index Array(array=w1238) -> (element #1=w1231:string, element #2=w1230:string, element #3=w1229:string, element #4=w1228:string, element #5=w1226:string, element #6=w1225:string, element #7=w1224:string, element #8=w1222:string, element #9=w1221:string, element #10=w1220:string)  [unwired: 10 in]
                n874 = Number To Decimal String(number=w1277) -> (decimal integer string=w1218:string)  [unwired: 1 in]
                n875 = Number To Decimal String(number=w1276) -> (decimal integer string=w1217:string)  [unwired: 1 in]
                n876 = Number To Decimal String(number=w1275) -> (decimal integer string=w1216:string)  [unwired: 1 in]
                n877 = Concatenate Strings(w1252, w1253, w1236, w1254, w1255, w1256, w1235, w1257, w1258, w1259, w1234, w1260, w1261, w1262, w1233, w1263, w1264, w1265, w1232, w1266, w1267, w1268, w1231, w1230, w1229, w1228, w1227, w1226, w1225, w1224, w1223, w1222, w1221, w1220, w1219, w1251, w1250, w1249, w1218, w1248, w1247, w1246, w1217, w1245, w1244, w1243, w1216) -> (w1215:string)
                n878 = local read "Expinfo name"() -> (w1271:string[])
                n879 = Increment(x=w1213) -> (x+1=w1214:i32)
                n880 = local write "Current test"(w1214) -> ()
                n881 = local read "File path"() -> (w1272:path)
                n882 = Index Array(array=w1271, index=w1213) -> (element=w1273:string)
                n883 = Build Path(base path=w1272, name or relative path=w1273) -> (appended path=w1269:path)
                n884 = Write to Text File(file (use dialog)=w1269, text=w1215, error in=w1270) -> (error out=w1274:errorcluster)  [unwired: 1 in, 2 out]
                n885 = call <vilib>:"Simple Error Handler.vi"("error in (no error)"=w1274) -> ()  [unwired: 4 in, 5 out]
              }
            }
          }
        }
        "iteration2" <- w820
      }
    }
    frame #4 {
      n886 = local write "End of test"(TRUE) -> ()
    }
  }
